vi "Doktorarbeit_Cornelius_1.73.vi"(0 "Heizer":refnum<visa-resource-name>="COM1", 1 "Setpoint\n START":bool, 2 "Write to File":bool, 3 "SP 1 shall be (°C)":dbl=20.0 min=0.0 max=999.0, 4 "Intervall (s)":u32=1 max=600, 5 "Write/\nRead":bool=TRUE, 6 "Delay (ms)":u32=500 min=100 max=600000, 7 "Auto Tune":bool, 9 "Standby":bool, 11 "Reset\nSTOPP":bool, 12 "Read Temperature":bool=TRUE, 13 "Get Values":bool, 15 "File Path":path) -> (8 "(°C)":dbl format="%#.3f", 14 "SP 1 is (°C)":dbl)   [LabVIEW 2010]
doc: "1. Verwendung\n\nDas Programm dient der Steuerung und Abfrage des Thermocontrollers I3252 und dem Auslesen von zwei VC 840 Messgeräten und einem Druckmessgerät Pfeiffer Single Gauge. \nDie Messgeräte werden Standardmäßig ausgelesen und erst nach Betätigung des Schalters \"Write to File\" in einer Textdatei abgespeichert. Das Eingabefeld \"Intervall\" legt den Abstand der Messpunkte fest.\nDer Setpoint für den Thermocontroller wird erst nach Betätigung des Tasters \"Setpoint START\" übernommen und angesteuert. Er wird ind den EEPROM des Gerätes geschrieben. Die Regelung kann mit Hilfe des Schalters \"Standby\" unterbrochen werden. Durch den Taster \"Reset STOPP\" kann der Setpoint aus dem EEPROM gelöscht werden.\nDie Eingabeflächen \"Constant\" und \"Thickness\" dienen der Berechnung des spezifischen Widerstands.\nDie Eingabeflächen \"User\" und \"Sample\" werden in den Header der Textdatei übernommen.\nDer Indikator \"File Path\" zeigt den aktuellen Speicherort der Textdatei an. Dieser wird nach ausschalten des Schalters \"Write to File\" gelöscht. Bei erneuten Schreiben muss ein neuer Speicherort gewählt werden. Bei Wahl desselben Speicherorts werden sämtliche bereits gespeicherte Daten gelöscht.\n\n\n2. Erläuterungen zum Blockdiagramm\n2.1 äußere Sequenz\nDie äußerte Sequenz besteht aus fünf Frames. Der erste dient der Initialisierung der Ports. Der zweite dient als Verzögerung um dem Programm genug Zeit zu geben die Ports zu öffnen. Jedoch senden die beiden VC 840 bereits Informationen an den Computer die in einem Puffer zwischengespeichert werden. Im dritten Frame wird dieser Puffer geleert. Somit kommt es zu keinem Framing Error. Desweiteren wird in diesem Frame die Startzeit der Messungen genommen. Im vierten Frame wird die eigentliche Messung und Verarbeitung der Daten durchgeführt. Die while-Schleife wird nur durch Auftreten eines Fehlers oder durch Betätigung des Stopbuttons auf dem Front Panel in der oberen linken Ecke unterbrochen. Im fünften und letzten Frame werden die Ports wieder geschlossen und beim Auftreten eines Fehlers wird das Programm automatisch gestoppt. Falls kein Fehler auftritt wird die Sequenz von vorne abgearbeitet.\n\n2.2 while-Schleife und innere Sequenz\n2.2.1 \"Event Structure\"\n2.2.1.1 Allgemein\nDer erste Frame beinhaltet ein \"Event Structure\". Dieser reagiert auf insgesamt elf verschiedene Ereignisse. Falls keines dieser Ereignisse auftreten sollte, warte die Struktur eine Millisekunde bevor die \"Event Structure\" verlassen wird. Die übrigen Ereignisse treten ein, wenn der entsprechende Kontroller eine Werteänderung erfährt.\n\n2.2.1.2 Event: Setpoint\nDieser Case besteht von außen nach innen aus einer Stacked Sequence, einer for-Loop und einer Flat Sequence die wiederum zwei \"Case Structures\" enthält. Als erstes wird bei dem Schalter \"Setpoint START\" der Blinkmodus aktiviert und bei dem Schalter \"Read Temperature\" deaktiviert. Danach folgt das eigentliche setzen des Temperatursollwerts. In der ersten Iteration wird dem Controller I3252 ein Schreibbefehl gesendet. Theoretisch kann der Setpoint in den RAM oder in den EEPROM geschrieben werden. Diese Auswahl erfolgt mit Hilfe des Schalters \"RAM\". Da das Schreiben in den RAM -Speicher aber aus diversen Gründen nicht erwünscht ist, wurde es nicht implementiert. Eine nachträgliche Implementierung ist aber leicht möglich, in dem die untere String-Konstante \"*P012\" durch \"*W012\" ersetzt wird. An diesem Befehl wird eine fünfstellige Hexadezimalzahl angehängt, die den Sollwert wiedergibt. Der Sollwert wird vorher mit zehn multipliziert, da das Komma standardmäßig nach der ersten Ziffer festgesetzt wurde (Bsp.: 800 wird gesendet um 80 einzustellen). Dieser Befehlsstrang wird an das Gerät mittels des SubVIs \"Comm_Interface\", auf welches später noch näher eingegangen wird, weitergegeben. Der durch das Gerät zurückgegebene String wird nicht verarbeitet.\nDie zweite Iteration dient dem Auslesen des eingestellten Sollwertes. Wahlweise kann der RAM- oder der EEPROM-Speicher ausgelesen werden. Die eigentliche Verarbeitung des Ausgabestrings erfolgt durch das SubVI \"Edit Setpoint\".\nDie Implementierung zur Einstellung des zweiten Setpoints erfolgt durch kopieren der ersten beiden Fälle und ersetzen der \"1\" im Befehf durch eine \"2\" (Bsp.: \"*P012\" zu \"*P022\"). Es darf aber nicht vergessen werden, dass dann ebenfalls die Anzahl der Iterationen angepasst werden muss.\nAls letztes wird der Blinkmodus des Schalters \"Setpoint START\" wieder deaktiviert.\n\n2.2.1.3 Event: Standby\nDieses Ereignis aktiviert bzw. deaktiviert als erstes den Blinckmodus des entsprechenden Schalters und sendet danach den Befehl zum aktivieren (\"*D03\") oder zum deaktivieren (\"*E03\") des Standbymodus an den Thermocontroller.\n\n2.2.1.4 Event: Set Command \nDer in das Feld \"Command shall be\" eingegebene Befehl wird an den Thermocontroller übermittlet. Die korrekte Form des Befehls ist im \"Communication Manuel\" nachzuschlagen. Das \"*\"-Zeichen wurde allerdings schon implementiert und muss somit nicht mit eingegeben werden.\n\n2.2.1.5 Event: Reset\nIn der ersten Iteration wird der Reset-Befehl an den Thermocontroller gesendet. In Folge wird der gesamte EEPROM-Speicher gelöscht. Deshalb wird in der zweiten Iteration der Setpoint aktualisiert. Dieser Befehl hat keinen Einfluss auf den RAM-Speicher. Die anschließende Wartezeit ist auf vier Sekunden festgesetzt und wurde empirisch ermittelt. Diese Zeit benötigt das Gerät um den Reset durchzuführen und für die Kommunikation wieder zur Verfügung zu stehen.\n\n2.2.1.6 Event: Auto Tune\nEs ist festgeschrieben, dass der Setpoint für die \"Auto Tune\"-Funktion wenigstens 20°C über der aktuellen Temperatur liegt. Deshalb wird zunächst der aktuelle Temperaturwert ausgelesen. Im zweiten Schritt werden zu diesem Wert zwanzig addiert und der Setpoint wird in den RAM-Speicher geschrieben. Das Schreiben in diesen Speicher ist nötig, da die \"Auto Tune\"-Funktion\" erst nach einem Reset startet. Im dritten Schritt wird der eigentliche Befehl für den \"Auto Tune\" gesendet (siehe dazu \"Communication Manuel\" S.27). Als vierte und letzte Iteration der for-Schleife folgt der bereits erwähnte Reset-Befehl. Der Temperatursollwert, der im RAM-Speicher eingetragen ist, muss zum Schluss wieder auf 0°C gesetzt werden. Die Zeit für die Ausführung des \"Auto Tune\"-Befehls wurde empirisch ermittelt und 45 s festgesetzt.\n\n2.2.1.7 Event: Write LOW/HI\nDieses Ereignis setzt die am Analogausgang anliegende Spannung fest. Normalerweise beträgt dieser Spannungswert 0-10 V. Das angeschlossene Netzteil verträgt aber maximal nur 2,3 V. Aus diesem Grund wird der \"%HIGH\" auf 23 gesetzt. Somit beträgt die maximal anliegende Spannung nur noch 23% von der maximal möglichen, d.h 2,3V. Ein niedrigerer Wert ist jederzeit möglich, genauso wie ein höherer für den Parameter \"%LOW\". Diese werden zunächst nacheinander in den RAM-Speicher geschrieben und anschließend wieder ausgelesen.\n\n2.2.1.8 Event: Set PID\nDie Werte für den PID-Regler können sowohl mit Hilfe der \"Auto Tune\"-Funktion, als auch manuell eingestellt werden. Es wird wiederum zwischen dem Schreiben in den RAM- und dem EEPROM-Speicher unterschieden. Zunächst werden die Werte für \"P\", \"I\" und \"D\", in dieser Reihenfolge, gesetzt und danach die aktuellen Werte ausgelesen.\n\n2.2.1.9 Event: Get Values\nDieses Ereignis hat zur Folge, dass die Werte für \"P\", \"I\", \"D\", \"%LOW\", \"%HIGH\" und des Setpoints wahlweise aus dem RAM- oder EEPROM-Speicher gelesen werden. Die aktuellen Werte werden nicht nur in die entsprechenden Anzeigefelder übernommen, sondern auch in die entsprechenden Eingabefelder, mit Ausnahme des Temperatursollwerts. \n\n2.2.1.10 Event: RAM\nPrinzipiell kann zwischen dem Schreiben in den RAM- oder EEPROM-Speicher des Thermocontrollers gewählt werden. Die entsprechende Schalterposition auf dem Frontpanel zeigt den aktuell verwendeten Speicher an. Die Anzeigewerte werden bei jedem Umschalten aktualisiert und sind im entsprechenden Speicher eingetragen. Die Implementierung ist identisch mit der des Ereignisses \"Get Values\". Es gilt zu beachten, dass die Werte für \"%LOW\" und \"%HIGH\" nur in den RAM-Speicher geschrieben werden können und somit auch nur aus diesem ausgelesen werden können.\n\n2.2.1.11 Event: Set Gauge to Zero\nMit Hilfe der SubVIs \"Get Pressure\" und \"Offset Display\" werden die Werte für den alten und den neuen Offset und der durch den zweiten Drucksensor ermittelt Druck ermittelt. \n\n2.2.1.12 Event: Write to File\nSollte der Schalter \"Write to File\" aktiviert werden, d.h. Schalterposition oben, so wird zunächst durch das SubVI \"Header\" ein Header für die unter \"File Path\" definierte Datei angelegt. Alle Werte, die bereits in der entsprechenden Datei stehen, werden dabei gelöscht.\n\n2.2.2 \"Timed Structures\"\nIm dritten Frame der inneren Sequenz werden die Werte für Zeitpunkt, Temperatur, Spannung, Strom und Druck ermittelt. Damit die Werte zum gleichen Zeitpunkt aufgenommen werden, werden \"Timed Sequences\" eingesetzt. Mit dem entsprechenden Schalter auf dem Front Panel unter dem Tab \"Settings\" kann gewählt werden, ob das entsprechende Gerät ausgelesen werden soll oder nicht. Die einzelnen Sequenzen werden parallel abgearbeitet, womit die Prozesszeit von diesem Frame durch der zeitintensivsten Sequenz abhängt. Dies ist in aller Regel das Auslesen der Temperatur, da ein \"Delay\" von 500 ms oder größer benötigt wird, um den Controller ordentlich ansprechen zu können.\nDie Systemzeit wird durch das SubVI \"System Time in Seconds\" in Sekunden umgerechnet und der in dem Parameter \"Starttime\" gespeicherte Wert wird abgezogen. Somit werden die Sekunden seit dem Start des Programms gezählt.\n\n2.2.3 restlichen Frames\nIm zweiten Frame wird das Intervall zwischen den einzelnen Messwerten festgelegt. Dabei wird der Wert des Parameters \"Delay\" abgezogen. Dieser Wert beträgt im Normalfall 500 ms und ist somit nicht vernachlääsigbar.\nDer Vierte Frame beinhaltet die Umrechnung des Temperatur-Strings in einen Temperaturwert durch das SubVI \"Edit Tmperature\", die Berechnung des spezifischen Widerstands durch das SubVI \"Resistivity Calculation\" und die Überprüfung des Druckwerts. Auch werden die neu gewonnen Werte in das entsprechende Shift-Register übernommen. Falls der Druckwert einen in dem Parameter \"Pressure Limit (mbar)\" festgelegten Grenzwert überschreiten sollte, wird der Thermocontroller automatisch in den Standby-Modus versetzt. Des Weiteren wird der Schalter \"Standby\" solange gesperrt, wie der Druck oberhalb des Grenzwertes liegt. Wenn der Druck wieder unter den Grenzwert gesunken ist, wird der Standby-Befehl nicht automatisch aufgehoben, sondern muss vom Benutzer durch Betätigung des entsprechenden Schalters gegeben werden.\nIm fünften Frame werden die Diagramme erstellt. Dabei wird jedes Mal von neuem das gesamte Shift-Register als Graph dargestellt. Weiterhin werden die Messwerte in ein 1D-Array geschrieben.\nDer sechste und letzte Frame beinhaltet den eigentlich Schreibvorgang der Messwerte in eine Textdatei und die Überprüfung ob ein Fehler vorliegt.\n\n2.3 SubVIs\n2.3.1 Allgemein\nDie SubVIs für die Messgeräte VC840 und das Druckmessgerät wurden aus anderen Quellen übernommen. \n\n2.3.2 \"Header\"\nIn den Header wird zunächst das aktuelle Datum und die aktuelle Zeit übernommen. Die ausgewählte Datei wird dabei überschrieben. Danach wird der Name des Benutzers und der Probe übernommen. Zum Schluss werden die Einheiten in einer Reihe, durch einen Tabulator getrennt, in den Header geschrieben.\n\n2.3.3 \"I3252 Comm Interface\"\nDieses VI stellt die Kommunikation mit dem Thermocontroller her und gibt den Ausgabe-String zurück.\n\n2.3.4 \"I3252 Edit Setpoint\"\nIm Ausgabe-String vom Thermocontroller ist an der vierten Stelle die Stelle des Dezimalpunktes verschlüsselt. Dieses Hexadezimalzahl wird herausgefiltert und an ein \"ENUM Controller\" übergeben. Dieser weist der Hexadezimalzahl eine Nummer zu, mit welcher ein Wert aus einem Array entnommen wird. Dieser Wert dient als Quotient. Der tatsächliche Wert kann somit errechnet werden.\n\n2.3.5 \"I3252 Edit Temperature\"\nDer Temperatur-String, der vom Thermocontroller zurückgegeben wird, wird in eine Dezimalzahl umgewandelt. Manchmal kommt es aus zu Dropouts, die durch dieses Programm herausgefiltert werden. Der letzte Wert wird dabei in einer \"Feedback Node\" gehalten unter der Annahme, dass sich der Temperaturwert nicht sprunghaft ändert.\n\n2.3.6 \"Resistivity Calculation\"\nDer spezifische Widerstand wird nach folgender Formel ausgerechnet. Dabei entspricht t der Dicke der Probe und C ist eine Konstante.\nrho=C*pi*t*U/(ln( 2)*I)\n\n2.3.7 \"System Time in Seconds\"\nZunächst wird die aktuelle Systemzeit ausgelesen. Danach wird diese in Stunden, Minuten und Sekunden aufgeteilt, alles in Sekunden umgerechnet und letztendlich addiert."
uses:
  <vilib>/Platform/TimedLoop/XDataNode/XDataNode.xnode
  <vilib>/Platform/TimedLoop/XDataNode/timing_clust.ctl
  <vilib>/Platform/TimedLoop/XDataNode/nitl_modes.ctl
  <vilib>/Platform/TimedLoop/XDataNode/wakeup.ctl
  <vilib>/Instr/_visa.llb/VISA Configure Serial Port (Instr).vi
  <vilib>/Platform/TimedLoop/scheduler/LVUserAPI/_suppVIs/Create_1kHz_TSource.vi
  <vilib>/Utility/file.llb/Write To Spreadsheet File (DBL).vi
  <vilib>/Platform/TimedLoop/XDataNode/XDNodeRunTimeDep.lvlib
  Labview 8 Tutorial/Dual Gauge/Dual Gauge.lvlib
panel:
  out "appended array":dbl[](array[numeric])
  in  "Tab Control":T1(tab)
  out "Pirani (VVP1 Scroll)":cluster{dbl[], dbl[]}(graph)
  in  "Thickness (nm)":dbl min=0.0
  in  "Constant":dbl=4.532 min=0.0 max=5.0
  in  "Sample":string
  in  "User":string
  out "Thermocouple (Sample holder 1)":cluster{dbl[], dbl[]}(graph)
  out "current time (s)":dbl
  out "data logger intervall (s)":dbl
  out "loop time (s)":dbl
  in  "stop":bool
  out "CMR275 Baratron":cluster{dbl[], dbl[]}(graph)
  out "Pressure Baratron 2":dbl format="%#_4e"
  out "PKR251 FullRange":cluster{dbl[], dbl[]}(graph)
  out "Pressure FullRange 2":dbl format="%#_3e"
  out "Pressure Pirani 2":dbl format="%#_3e"
  out "Pressure OpenPort":cluster{dbl[], dbl[]}(graph)
  out "Pressure OpenPort2":dbl caption="current"
  out "Current Baratron (mbar)":dbl
  out "Error COM6 Out":cluster{"status":bool, "code":i32} caption="Cluster (Ausgang)"
  out "Pressure Pirani":dbl format="%.3e"
  out "Pressure OpenPort":dbl format="%.3e"
  out "Status Sensor 4":i32(ring) items=["data OK", "underrange", "overrange", "sensor error", "sensor off", "no sensor", "ID error"]
  out "Status Pirani":i32(ring) items=["data OK", "underrange", "overrange", "sensor error", "sensor off", "no sensor", "ID error"]
  in  "COM6 in":refnum<visa-resource-name>="COM6"
  out "Error COM5 Out":cluster{"status":bool, "code":i32} caption="Cluster (Ausgang)"
  out "Pressure FullRange":dbl format="%.3e"
  out "Pressure Baratron":dbl format="%.3e"
  out "Status FullRange":i32(ring) items=["data OK", "underrange", "overrange", "sensor error", "sensor off", "no sensor", "ID error"]
  out "Status Baratron":i32(ring) items=["data OK", "underrange", "overrange", "sensor error", "sensor off", "no sensor", "ID error"]
  in  "COM5 in":refnum<visa-resource-name>="COM5"
  out "Error Out":bool
  in  "Set Gauge to Zero":bool
  in  "Pressure Limit (mbar)":dbl=1.0 min=0.0 max=1100.0
  out "Current Offset (mbar)":dbl
  out "Old Offset (mbar)":dbl
  out "Pressure 2 (mbar)":dbl
  in  "VC 840 2":refnum<visa-resource-name>="COM7"
  out "Reading 2":dbl format="%_4f"
  out "Mode 2":enum16{"?", "Diode", "Beep", "DC", "AC"}(ring)
  out "Unit 2":string
  in  "VC 840 1":refnum<visa-resource-name>="COM7"
  out "Reading 1":dbl format="%_4f"
  out "Mode 1":enum16{"?", "Diode", "Beep", "DC", "AC"}(ring)
  out "Unit 1":string
  out "Status 1":T2
  out "Status 2":T2
  in  "Read VC 840 1":bool
  in  "Read VC 840 2":bool
  in  "Set Command":bool
  in  "Set PID":bool
  in  "Write LOW/HI":bool
  out "% HIGH is":u32
  out "% LOW is":u32
  in  "% High shall be":u32=23 max=24
  in  "% LOW shall be":u32 max=25
  in  "Flow Control":u16(ring) items=["None"=0, "XON/XOFF"=1, "RTS/CTS"=2, "DTR/DSR"=4]
  in  "Stop Bits":u16(ring)=10 items=["1.0"=10, "1.5"=15, "2.0"=20]
  in  "Parity":u16(ring)=1 items=["None", "Odd", "Even", "Mark", "Space"]
  in  "Data Bits":u16=7 min=5 max=8 step=1
  in  "Baud Rate":u32=9600
  out "Command is":string
  in  "Command shall be":string
  in  "RAM":bool=TRUE caption="EEPROM"
  out "D (Rate) is":u32
  out "I ( Reset1) is":u32
  out "P (PB1) is":u32
  in  "D (Rate) shall be":u32 max=3999
  in  "I ( Reset1) shall be":u32 max=3999
  in  "P (PB1) shall be":u32 max=9999
  in  "Read Pressure":bool=TRUE
  out "Current":cluster{dbl[], dbl[]}(graph)
  out "Voltage":cluster{dbl[], dbl[]}(graph)
  out "Voltage (V)":dbl format="%.4e"
  out "Current (A)":dbl format="%.4e"
  out "Resistivity":cluster{dbl[], dbl[]}(graph)
  out "Resistivity (Ohm*cm)":dbl format="%.3e"
  # "°C"
  # "mbar"
  # "mbar"
  # "mbar"
  # "mbar"
  # "Offset Control"
  # "Sensor Diagnose"
  # "mbar"
  # "mbar"
  # "mbar"
  # "mbar"
  # "VC 840 Control"
  # "I3252 Control"
  # "Pfeiffer Control"
  # "Authors:  Daniel Schuster (sir-dan@web.de)\n                 Steffen Cornelius (s.cornelius@hzdr.de)\n                 Nico Spahn (x)\n\n                 premade SubVIs for readout of Pfeiffer gauge and VC840 Multimeters were used\n                 SubVI \"I3252_Comm_Interface\" is based on a modified Labview example\n\nRelease:  v1.0    \n\nVersion History:\n\nv1.1  -    28.06.2011\n             - Format des Files geändert von %.3f auf %g\n             - maximale Eingabewerte für PID begrenzt\nv1.2  -    12.07.2011\n             - Anzeige p,rho, U, V auf Scientific geändert\n             - y-Achse p,rho auf Log geändert\n             - numerische Zeitanzeige hinzugefügt\n             - 4PP Constant: pi/ln(2)=4,532 set as the default value\nv1.3  -    25.07.2011\n             - Zeitvariable auf EXT geändert, um Sprünge in Diagrammen loszuwerden\nv1.4  -   27.07.2011\n             - ALLE Variablen auf DBL zurückgesetzt wegen Formatierungsproblem im File\n             - Zeitberechnung neu gemacht (Tick count differenzen) -> Zeitsprünge korrigiert ?\n             - Delay/Intervall überarbeitet\nv1.5  -   05.12.2012\n                - Austausch der alten Pfeifer SubvIs durch neue -> nun alle 4 Kanäle des DualGauge\n                                                                                                         Controllers gleichzeitig auslesbar\n                - neue Pfeiffer SubVIs verwendet in Druckwertauslesung und Offset Berechnung des Baratron\n                  Druckes (COM5 Sensor1)\n                - Neuarragement des GUI -> FullRange und Baratron neben Temperatur auf Haupseite zu sehen\n                                                                   Pirani und OpenPort auf Meas.2 zu sehen\n                                                                   Diagnose Seite umfasst nun auch Widerstandsdiagramm\n                - Änderungen der Settingseite -> nun alle 4 Drucksensoren mit aktuellem Messwert und Gerätestatus\n                                                                           zu sehen\n                - The readout of the PID-Temperature Controller and the VC840 Multimeters was not modified\nv1.73  -  18.10.2013\n                - Layout Änderungen"
  # "Version 1.73    - last change 18.10.2013"
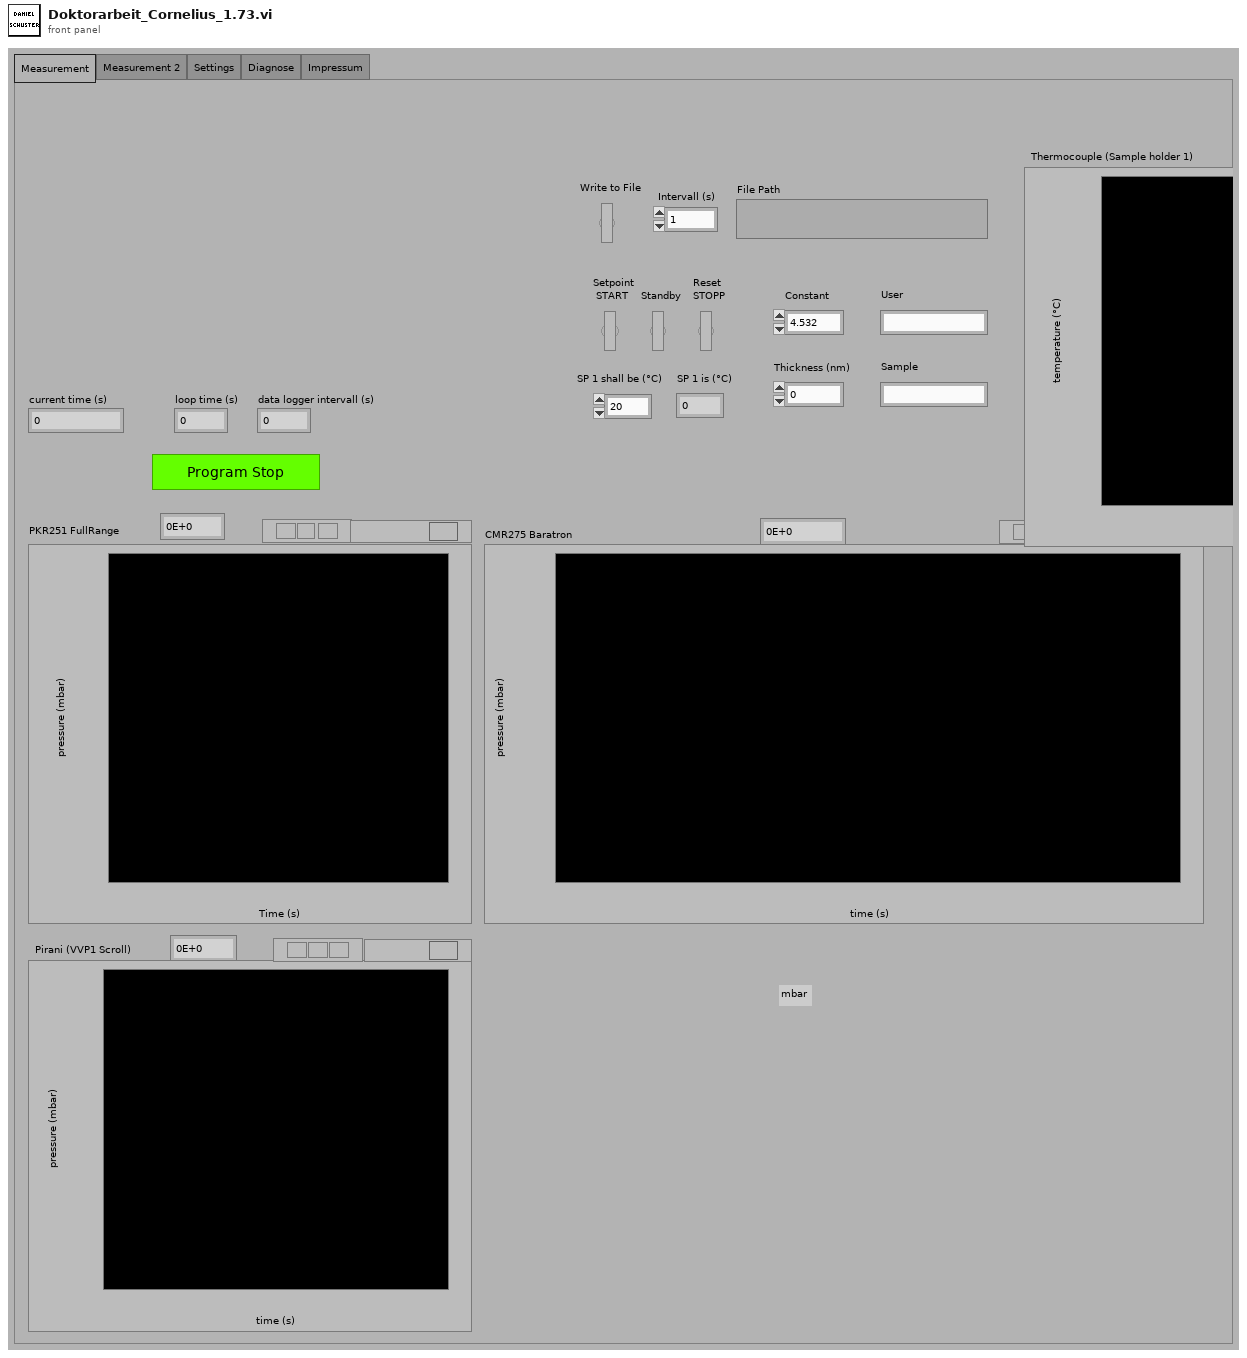
[diagram p1: front panel]
types:
  T1 = enum32{"Measurement", "Measurement 2", "Settings", "Diagnose", "Impressum"}
  T2 = cluster{"Low Bat":bool, "Auto":bool, "Delta":bool, "Hold":bool, "RS232":bool}
  T3 = typedef "XDNodeRunTimeDep.lvlib/timing_clust.ctl" = cluster{"Expected End [f-1]":u64, "Actual End [f-1]":u64, "Finished Late? [f-1]":bool, "Expected End [i-1]":u64, "Actual End [i-1]":u64, "Finished Late? [i-1]":bool, "Expected Start [i]":u64, "Actual Start [i]":u64, "Expected Start [f]":u64, "Actual Start [f]":u64, "Source Name":string, "Structure Name":string, "Period":i64, "Deadline":i64, "Offset":i64, "Start":i64, "Priority":i32, "Timeout":i32, "Mode":T4, "Wakeup Reason":T5, "Error":errorcluster, "Source Type":string, "Secondary Source Type":string, "Global End Time":u64, "Global Start Time":u64, "Frame Duration":u64, "Iteration Duration":u64, "Assigned CPU":i32, "I/O Scan Engine Mode":u32}
  T4 = typedef "XDNodeRunTimeDep.lvlib/nitl_modes.ctl" = enum32{"No Change", "Process missed periods, maintain original phase", "Discard missed periods, maintain original phase", "Process missed periods, ignore original phase", "Discard missed periods, ignore original phase"}
  T5 = typedef "XDNodeRunTimeDep.lvlib/wakeup.ctl" = enum32{"Normal", "Aborted", "Asynchronous wakeup", "Timing source error", "Timed loop error", "Timeout"}
  T6 = enum8{"Enabled", "Disabled", "Disabled and Grayed Out"}
  T7 = cluster{"VISA resource name out":refnum<visa-resource-name>, "error out":errorcluster, "Delay (ms)":u32, "Write/\nRead":bool}
  T8 = cluster{"Pressure":dbl, "Pressure":dbl, "Pressure":dbl, "Pressure":dbl}
  T9 = cluster{"COM5 in":refnum<visa-resource-name>, "error out":errorcluster, "COM6 in":refnum<visa-resource-name>, "error out":errorcluster}
  T10 = cluster{"COM5 out":refnum<visa-resource-name>, "Cluster (Ausgang)":errorcluster, "COM6 out":refnum<visa-resource-name>, "Cluster (Ausgang) 2":errorcluster}
  T11 = cluster{"Pressure Baratron":dbl, "Pressure FullRange":dbl, "Pressure Pirani":dbl, "Pressure Sensor 4":dbl}
  T12 = cluster{"COM5 out":refnum<visa-resource-name>, "error out":errorcluster, "COM6 out":refnum<visa-resource-name>, "error out":errorcluster}
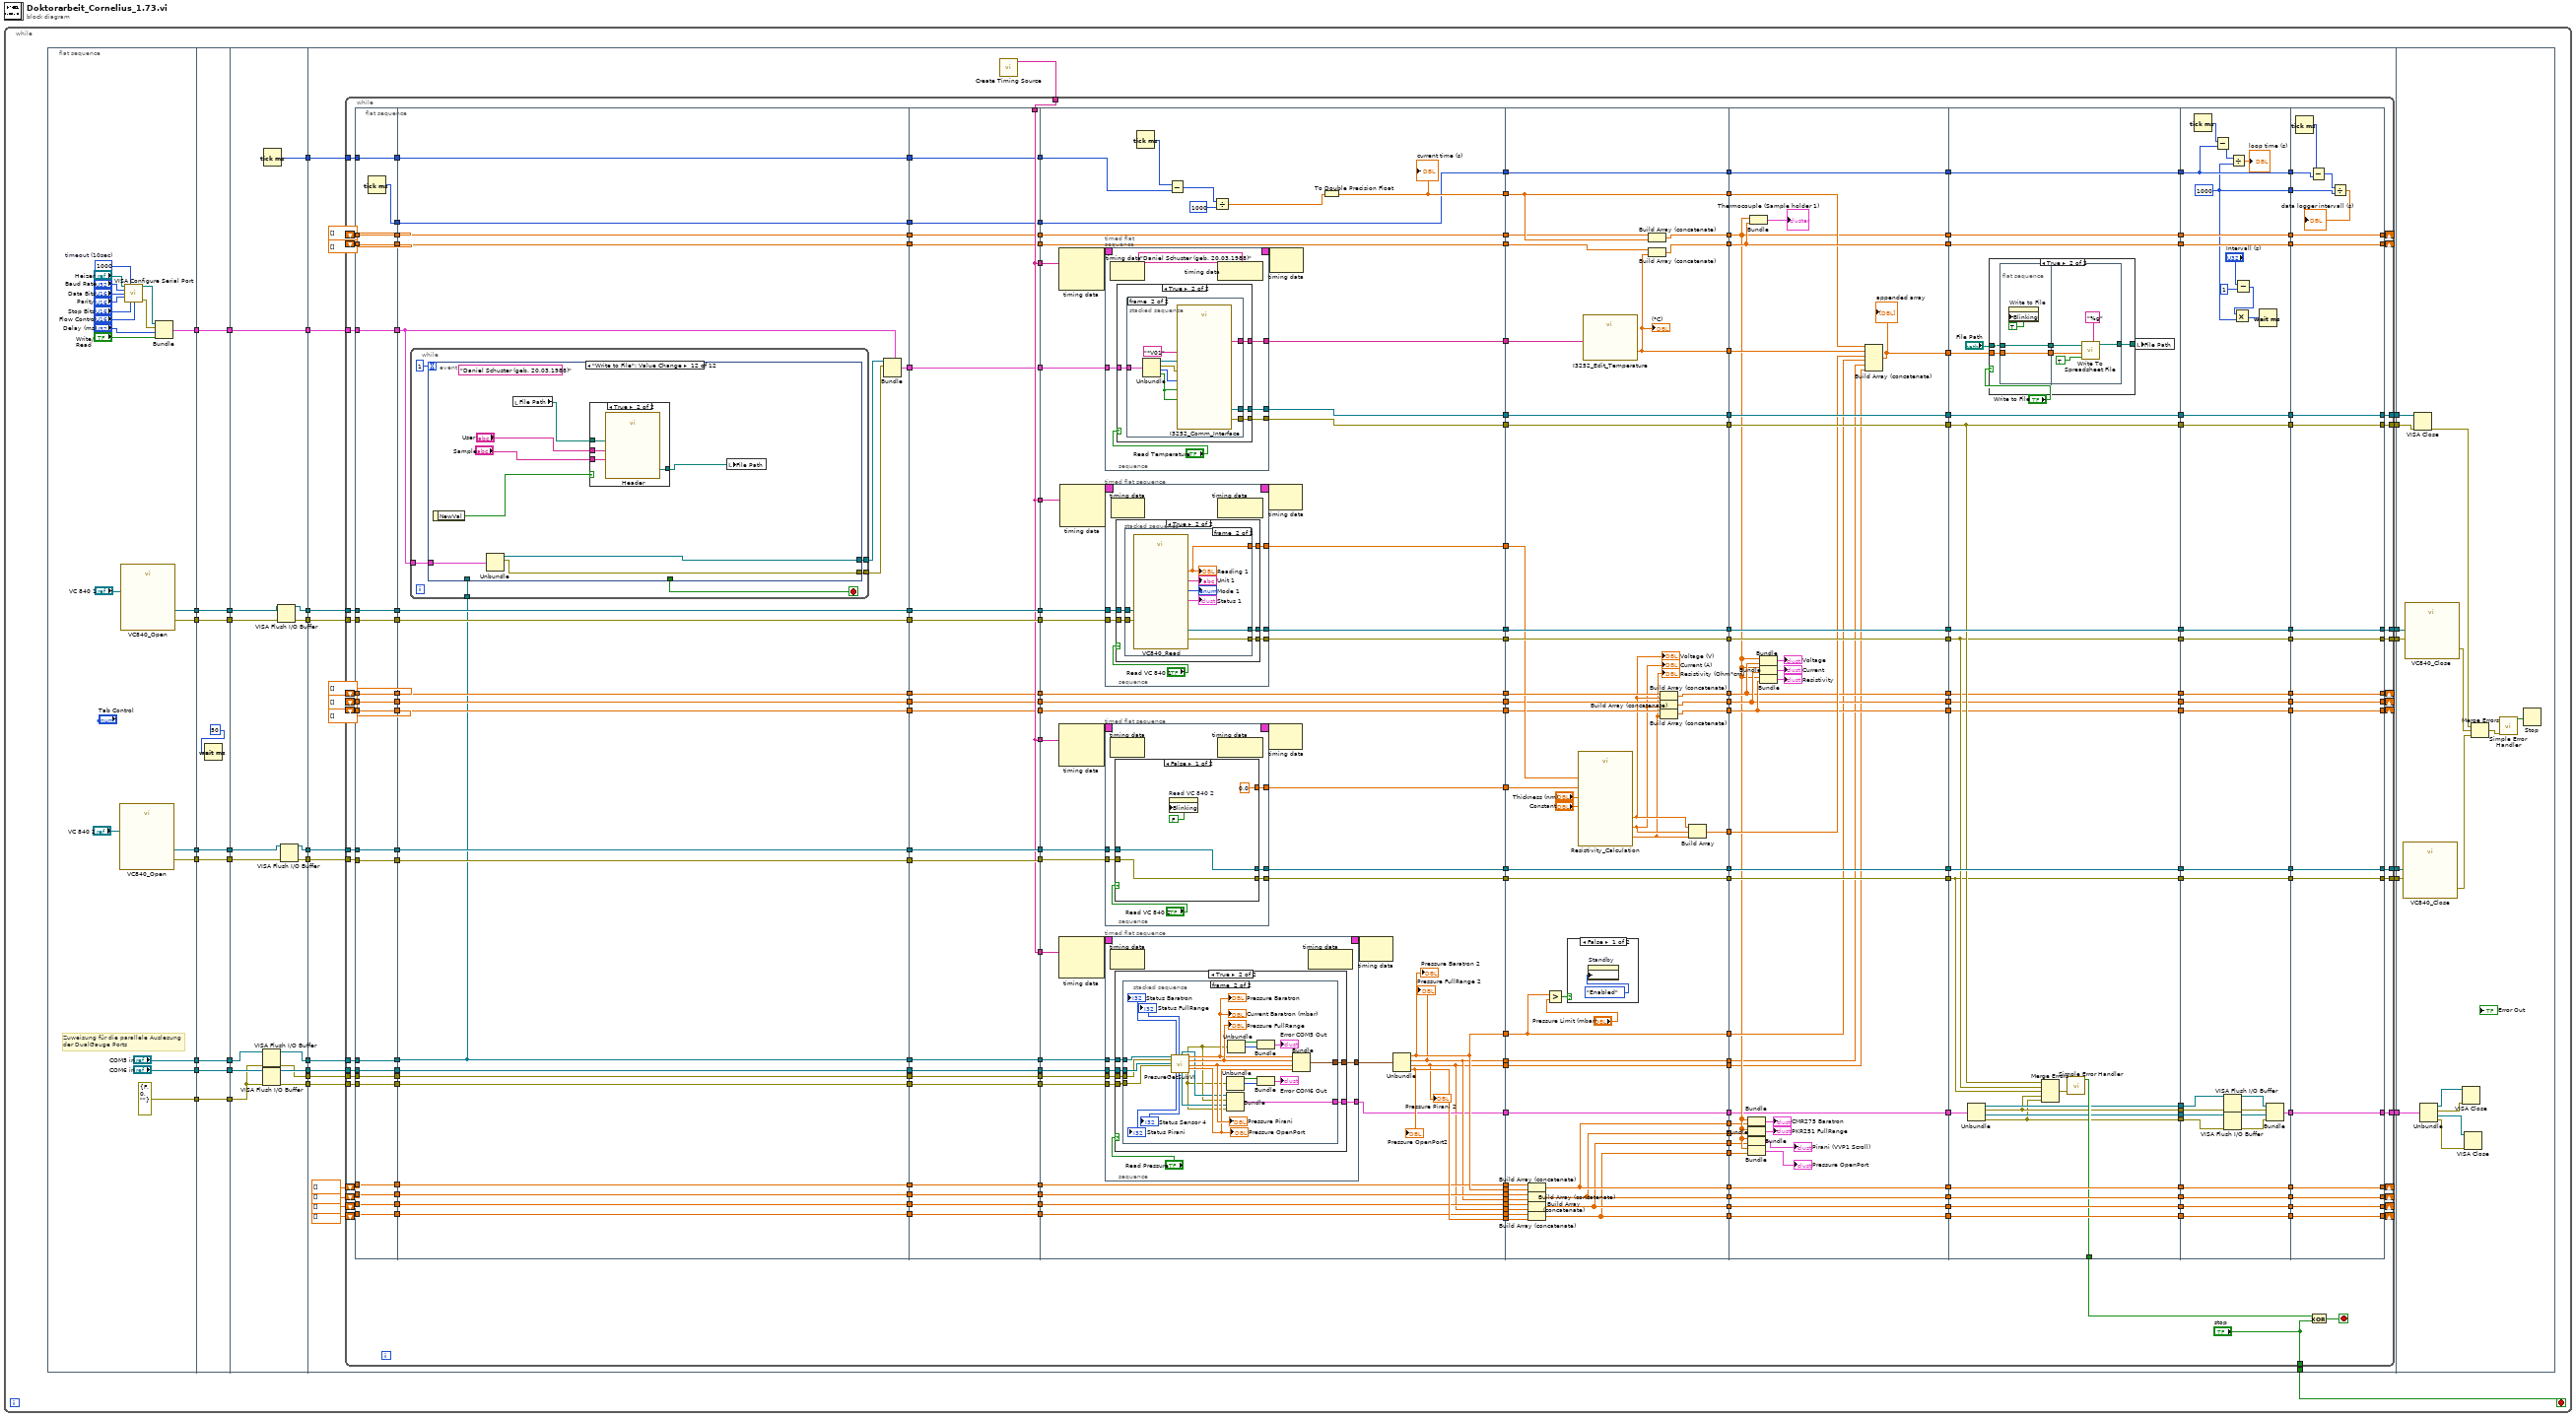
[diagram p0: block diagram]
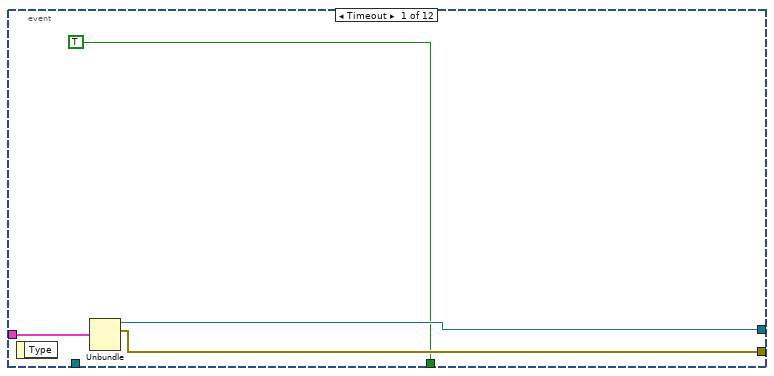
[diagram p2: hidden frame]
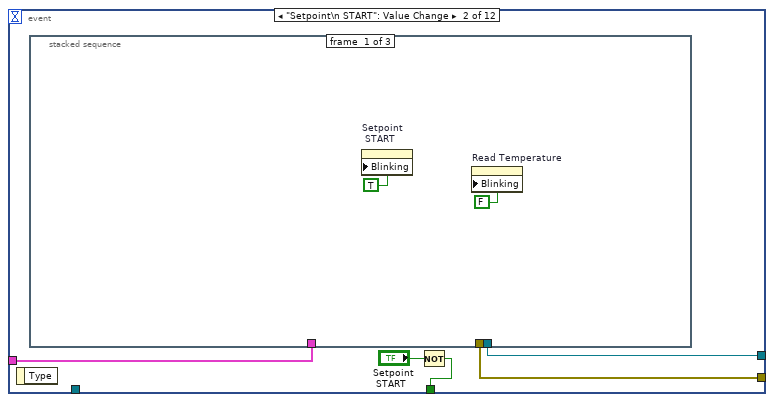
[diagram p3: hidden frame]
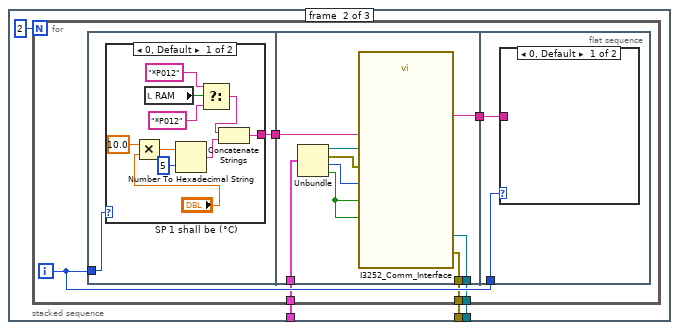
[diagram p4: hidden frame]
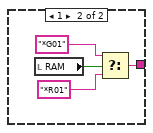
[diagram p5: hidden frame]
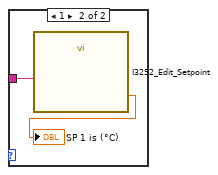
[diagram p6: hidden frame]
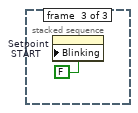
[diagram p7: hidden frame]
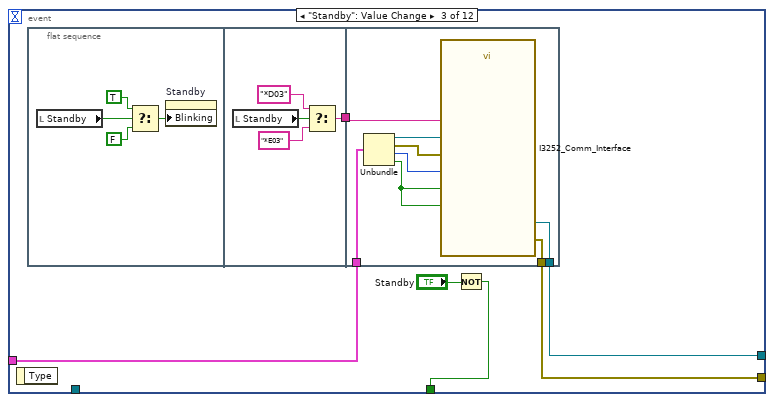
[diagram p8: hidden frame]
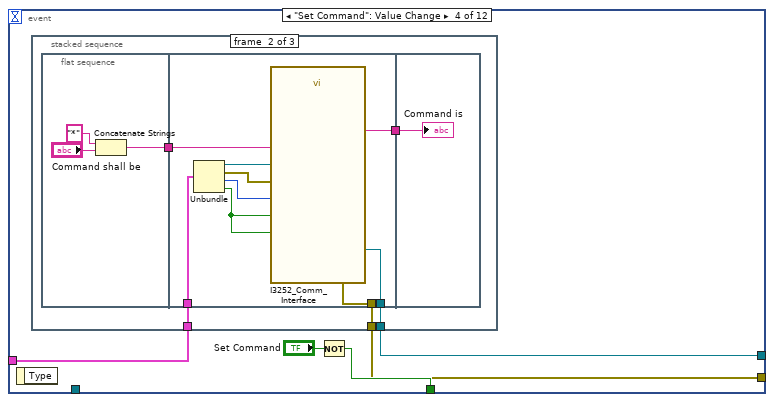
[diagram p9: hidden frame]
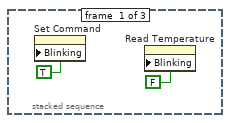
[diagram p10: hidden frame]
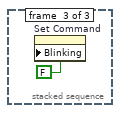
[diagram p11: hidden frame]
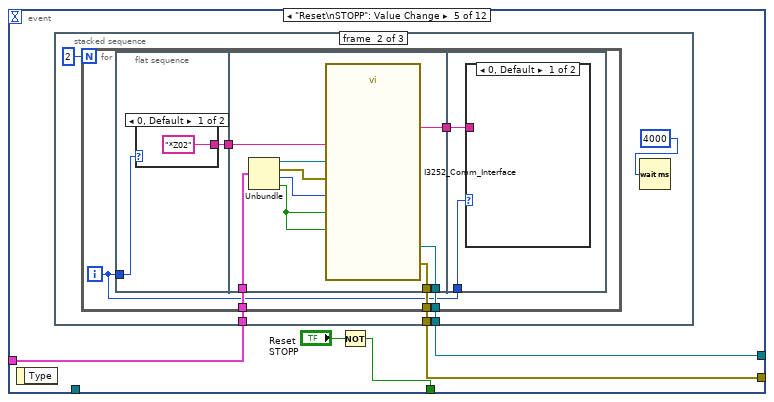
[diagram p12: hidden frame]
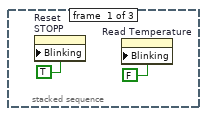
[diagram p13: hidden frame]
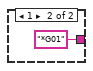
[diagram p14: hidden frame]
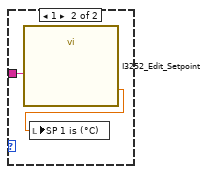
[diagram p15: hidden frame]
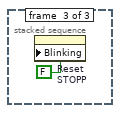
[diagram p16: hidden frame]
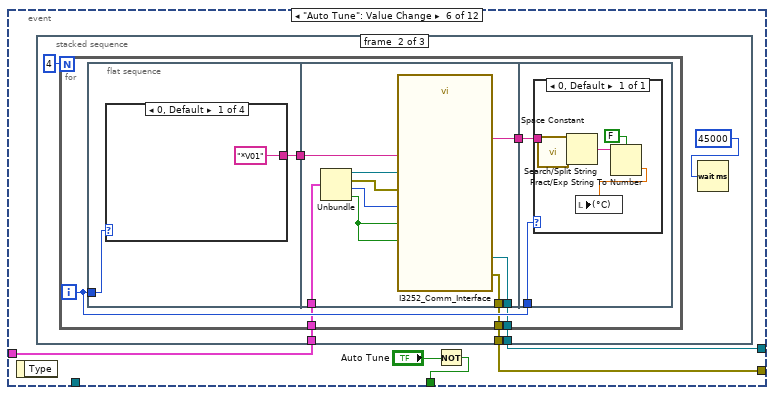
[diagram p17: hidden frame]
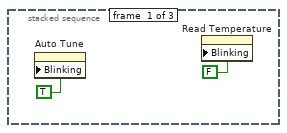
[diagram p18: hidden frame]
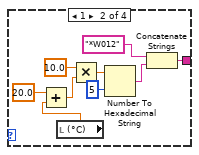
[diagram p19: hidden frame]
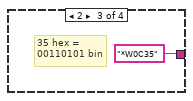
[diagram p20: hidden frame]
diagram:
  n1 = while {
    stop <- w6 stop-if-true
    n2 = flat-sequence {
      tunnel: [w54] -> w34
      tunnel: [w55] -> w33
      tunnel: [w40] -> w32
      tunnel: [w53] -> w31
      tunnel: [w52] -> w30
      tunnel: ["COM5 in"] -> w29
      tunnel: ["COM6 in"] -> w28
      tunnel: [errorcluster {"status"=FALSE, "code"=0, "source"=""} ("Fehler (Eingang)")] -> w3
      tunnel: w34 -> [w64]
      tunnel: [w64] -> w27
      tunnel: w33 -> [w63]
      tunnel: [w63] -> w26
      tunnel: w32 -> [w62]
      tunnel: [w62] -> w25
      tunnel: w31 -> [w61]
      tunnel: [w61] -> w24
      tunnel: w30 -> [w60]
      tunnel: [w60] -> w23
      tunnel: [w58] -> w22
      tunnel: w29 -> [w58]
      tunnel: [w57] -> w21
      tunnel: w28 -> [w57]
      tunnel: [w56] -> w4
      tunnel: w3 -> [w56]
      tunnel: w27 -> [w75]
      tunnel: [w74] -> w20
      tunnel: w26 -> [w76]
      tunnel: [w73] -> w19
      tunnel: w25 -> [w81]
      tunnel: [w81] -> w18
      tunnel: w24 -> [w78]
      tunnel: [w79] -> w17
      tunnel: w23 -> [w77]
      tunnel: [w80] -> w16
      tunnel: [w72] -> w15
      tunnel: [w70] -> w14
      tunnel: w22 -> [w71]
      tunnel: [w69] -> w13
      tunnel: w21 -> [w68]
      tunnel: w4 -> [w67]
      tunnel: [w66] -> w2
      tunnel: [w65] -> w1
      tunnel: w20 -> [w109]
      tunnel: w19 -> [w108]
      tunnel: w18 -> [w107]
      tunnel: w17 -> [w105]
      tunnel: w16 -> [w104]
      tunnel: [w103] -> w12
      tunnel: [w102] -> w11
      tunnel: [w101] -> w10
      tunnel: [w100] -> w9
      tunnel: [w99] -> w8
      tunnel: [w98] -> w7
      tunnel: w15 -> [w92]
      tunnel: w14 -> [w91]
      tunnel: w13 -> [w90]
      tunnel: [w85] -> w6
      tunnel: [w84] -> w5
      tunnel: w2 -> [w83]
      tunnel: w1 -> [w82]
      tunnel: w12 -> [w1292]
      tunnel: w11 -> [w1291]
      tunnel: w10 -> [w1294]
      tunnel: w9 -> [w1293]
      tunnel: w8 -> [w1296]
      tunnel: w7 -> [w1295]
      tunnel: w5 -> [w1289]
      frame #0 {
        w41 = u32 1000  # timeout (10sec)
        # "Zuweisung für die parallele Auslesung\nder DualGauge Ports"
        n3 = call "VC840_Open.vi"("VISA resource name"="VC 840 2") -> ("error out"=w52:errorcluster, "VISA resource name out"=w53:refnum<visa-resource-name>)  [unwired: 1 in, 8 out]
        n4 = call "VC840_Open.vi"("VISA resource name"="VC 840 1") -> ("error out"=w55:errorcluster, "VISA resource name out"=w54:refnum<visa-resource-name>)  [unwired: 1 in, 8 out]
        n5 = call-poly "VISA Configure Serial Port"("VISA resource name"="Heizer", "timeout (10sec)"=w41, "baud rate (9600)"="Baud Rate", "data bits (8)"="Data Bits", "parity (0:none)"="Parity", "stop bits (10: 1 bit)"="Stop Bits", "flow control (0:none)"="Flow Control") -> ("VISA resource name out"=w50:refnum<visa-resource-name>, "error out"=w51:errorcluster)  [unwired: 2 in, 5 out]
        n6 = Bundle("VISA resource name out"=w50, "error out"=w51, "Delay (ms)"="Delay (ms)", "Write/\nRead"="Write/\nRead") -> (w40:T7)  [unwired: 1 in]
      }
      frame #1 {
        n7 = Wait (ms)(milliseconds to wait=u32 50) -> ()  [unwired: 1 out]
      }
      frame #2 {
        n8 = VISA Flush I/O Buffer(VISA resource name=w71, error in (no error)=w67) -> (VISA resource name out=w70:refnum<visa-resource-name>, error out=w66:errorcluster)  [unwired: 1 in]
        n9 = VISA Flush I/O Buffer(VISA resource name=w68, error in (no error)=w67) -> (VISA resource name out=w69:refnum<visa-resource-name>, error out=w65:errorcluster)  [unwired: 1 in]
        n10 = Tick Count (ms)() -> (millisecond timer value=w72:u32)
        n11 = VISA Flush I/O Buffer(VISA resource name=w75, error in (no error)=w76) -> (VISA resource name out=w74:refnum<visa-resource-name>, error out=w73:errorcluster)  [unwired: 1 in]
        n12 = VISA Flush I/O Buffer(VISA resource name=w78, error in (no error)=w77) -> (VISA resource name out=w79:refnum<visa-resource-name>, error out=w80:errorcluster)  [unwired: 1 in]
      }
      frame #3 {
        n13 = call-poly <vilib>:"Create Timing Source.vi"() -> ("name (out)"=w106:string)  [unwired: 10 in, 1 out]
        n14 = while {
          tunnel: w109 -> [w323]
          tunnel: w108 -> [w322]
          tunnel: w107 -> [w321]
          tunnel: w106 -> [w314]
          tunnel: w105 -> [w307]
          tunnel: w104 -> [w306]
          tunnel: [w302] -> w103
          tunnel: [w301] -> w102
          tunnel: [w299] -> w101
          tunnel: [w297] -> w100
          tunnel: [w295] -> w99
          tunnel: [w293] -> w98
          shift-right: [w266] -> _
          shift-left: dbl[] [] -> [w271]
          shift-right: [w244] -> _
          shift-left: dbl[] [] -> [w279]
          shift-right: [w268] -> _
          shift-left: dbl[] [] -> [w275]
          shift-right: [w241] -> _
          shift-left: dbl[] [] -> [w278]
          shift-right: [w238] -> _
          shift-left: dbl[] [] -> [w277]
          tunnel: w92 -> [w232]
          tunnel: w91 -> [w188]
          tunnel: w90 -> [w184]
          shift-right: [w140] -> _
          shift-left: dbl[] [] -> [w170]
          shift-right: [w138] -> _
          shift-left: dbl[] [] -> [w168]
          shift-right: [w136] -> _
          shift-left: dbl[] [] -> [w166]
          shift-right: [w134] -> _
          shift-left: dbl[] [] -> [w164]
          tunnel: ["stop"] -> w85
          tunnel: [w126] -> w84
          tunnel: w83 -> [w121]
          tunnel: w82 -> [w119]
          stop <- w125 stop-if-true
          n15 = flat-sequence {
            tunnel: w232 -> [w333]
            tunnel: w271 -> [w334]
            tunnel: w275 -> [w335]
            tunnel: w277 -> [w336]
            tunnel: w278 -> [w337]
            tunnel: w279 -> [w338]
            tunnel: w306 -> [w339]
            tunnel: w307 -> [w340]
            tunnel: w321 -> [w341]
            tunnel: w322 -> [w342]
            tunnel: w323 -> [w343]
            tunnel: [w343] -> w231
            tunnel: [w342] -> w230
            tunnel: [w341] -> w229
            tunnel: [w340] -> w228
            tunnel: [w339] -> w227
            tunnel: [w338] -> w226
            tunnel: [w337] -> w225
            tunnel: [w336] -> w224
            tunnel: [w335] -> w223
            tunnel: [w334] -> w222
            tunnel: [w333] -> w221
            tunnel: [w332] -> w203
            tunnel: [w331] -> w189
            tunnel: w188 -> [w331]
            tunnel: [w330] -> w185
            tunnel: w184 -> [w330]
            tunnel: [w329] -> w171
            tunnel: w170 -> [w329]
            tunnel: [w328] -> w169
            tunnel: w168 -> [w328]
            tunnel: [w327] -> w167
            tunnel: w166 -> [w327]
            tunnel: [w326] -> w165
            tunnel: w164 -> [w326]
            tunnel: [w325] -> w122
            tunnel: w121 -> [w325]
            tunnel: [w324] -> w120
            tunnel: w119 -> [w324]
            tunnel: [w366] -> w320
            tunnel: [w365] -> w318
            tunnel: [w361] -> w316
            tunnel: [w360] -> w311
            tunnel: [w359] -> w309
            tunnel: [w358] -> w276
            tunnel: [w357] -> w272
            tunnel: [w356] -> w252
            tunnel: [w355] -> w249
            tunnel: [w354] -> w247
            tunnel: [w353] -> w233
            tunnel: w231 -> [w366]
            tunnel: w230 -> [w365]
            tunnel: w229 -> [w364]
            tunnel: w228 -> [w360]
            tunnel: w227 -> [w359]
            tunnel: w226 -> [w356]
            tunnel: w225 -> [w355]
            tunnel: w224 -> [w354]
            tunnel: w223 -> [w358]
            tunnel: w222 -> [w357]
            tunnel: w221 -> [w353]
            tunnel: [w352] -> w204
            tunnel: w203 -> [w352]
            tunnel: w189 -> [w350]
            tunnel: [w350] -> w186
            tunnel: w185 -> [w351]
            tunnel: [w351] -> w182
            tunnel: w171 -> [w349]
            tunnel: w169 -> [w348]
            tunnel: w167 -> [w347]
            tunnel: w165 -> [w346]
            tunnel: [w349] -> w163
            tunnel: [w348] -> w159
            tunnel: [w347] -> w156
            tunnel: [w346] -> w155
            tunnel: w122 -> [w345]
            tunnel: w120 -> [w344]
            tunnel: [w345] -> w117
            tunnel: [w344] -> w115
            tunnel: w320 -> [w891]
            tunnel: [w891] -> w319
            tunnel: w318 -> [w890]
            tunnel: [w890] -> w317
            tunnel: w316 -> [w886]
            tunnel: [w886] -> w315
            tunnel: w314 -> [w887]
            tunnel: [w887] -> w313
            tunnel: [w887] -> w312
            tunnel: w311 -> [w889]
            tunnel: [w889] -> w310
            tunnel: w309 -> [w888]
            tunnel: [w888] -> w308
            tunnel: [w887] -> w305
            tunnel: [w887] -> w291
            tunnel: w276 -> [w885]
            tunnel: [w885] -> w274
            tunnel: w272 -> [w884]
            tunnel: [w884] -> w269
            tunnel: [w883] -> w253
            tunnel: w252 -> [w883]
            tunnel: [w882] -> w250
            tunnel: w249 -> [w882]
            tunnel: [w881] -> w248
            tunnel: w247 -> [w881]
            tunnel: [w880] -> w234
            tunnel: w233 -> [w880]
            tunnel: [w879] -> w205
            tunnel: w204 -> [w879]
            tunnel: [w878] -> w187
            tunnel: w186 -> [w878]
            tunnel: [w877] -> w183
            tunnel: w182 -> [w877]
            tunnel: w163 -> [w876]
            tunnel: [w876] -> w162
            tunnel: [w875] -> w160
            tunnel: w159 -> [w875]
            tunnel: [w874] -> w158
            tunnel: w156 -> [w874]
            tunnel: w155 -> [w873]
            tunnel: [w873] -> w154
            tunnel: [w872] -> w118
            tunnel: w117 -> [w872]
            tunnel: [w871] -> w116
            tunnel: w115 -> [w871]
            tunnel: [w912] -> w290
            tunnel: w319 -> [w941]
            tunnel: w317 -> [w940]
            tunnel: w315 -> [w937]
            tunnel: w313 -> [w936]
            tunnel: w312 -> [w935]
            tunnel: w310 -> [w925]
            tunnel: w308 -> [w924]
            tunnel: w305 -> [w926]
            tunnel: [w922] -> w289
            tunnel: [w923] -> w288
            tunnel: [w934] -> w287
            tunnel: [w933] -> w286
            tunnel: [w932] -> w285
            tunnel: [w931] -> w284
            tunnel: w291 -> [w921]
            tunnel: [w920] -> w283
            tunnel: [w919] -> w282
            tunnel: [w902] -> w281
            tunnel: [w918] -> w280
            tunnel: w274 -> [w917]
            tunnel: [w917] -> w273
            tunnel: [w916] -> w270
            tunnel: w269 -> [w916]
            tunnel: w253 -> [w915]
            tunnel: [w915] -> w251
            tunnel: w250 -> [w914]
            tunnel: w248 -> [w913]
            tunnel: [w914] -> w246
            tunnel: [w913] -> w245
            tunnel: w234 -> [w911]
            tunnel: [w907] -> w206
            tunnel: w205 -> [w907]
            tunnel: w187 -> [w905]
            tunnel: w183 -> [w904]
            tunnel: [w896] -> w181
            tunnel: [w902] -> w180
            tunnel: [w892] -> w179
            tunnel: [w901] -> w178
            tunnel: [w899] -> w177
            tunnel: [w897] -> w176
            tunnel: w162 -> [w900]
            tunnel: [w900] -> w161
            tunnel: w160 -> [w899]
            tunnel: w158 -> [w898]
            tunnel: [w898] -> w157
            tunnel: w154 -> [w897]
            tunnel: [w896] -> w132
            tunnel: [w892] -> w130
            tunnel: [w895] -> w127
            tunnel: w118 -> [w894]
            tunnel: w116 -> [w893]
            tunnel: w290 -> [w1137]
            tunnel: [w1134] -> w264
            tunnel: w289 -> [w1150]
            tunnel: [w1150] -> w263
            tunnel: w288 -> [w1149]
            tunnel: [w1149] -> w262
            tunnel: w287 -> [w1148]
            tunnel: [w1148] -> w261
            tunnel: w286 -> [w1147]
            tunnel: [w1147] -> w260
            tunnel: w285 -> [w1146]
            tunnel: [w1146] -> w259
            tunnel: w284 -> [w1145]
            tunnel: [w1145] -> w258
            tunnel: [w1138] -> w257
            tunnel: w283 -> [w1131]
            tunnel: w282 -> [w1139]
            tunnel: w281 -> [w1138]
            tunnel: w280 -> [w1140]
            tunnel: [w1137] -> w256
            tunnel: w273 -> [w1136]
            tunnel: w270 -> [w1135]
            tunnel: [w1133] -> w255
            tunnel: [w1121] -> w254
            tunnel: w251 -> [w1132]
            tunnel: w246 -> [w1129]
            tunnel: w245 -> [w1128]
            tunnel: [w1130] -> w242
            tunnel: [w1127] -> w239
            tunnel: [w1126] -> w236
            tunnel: [w1122] -> w235
            tunnel: [w1120] -> w207
            tunnel: w206 -> [w1120]
            tunnel: w181 -> [w1119]
            tunnel: w180 -> [w1118]
            tunnel: w179 -> [w1117]
            tunnel: w178 -> [w1116]
            tunnel: w177 -> [w1115]
            tunnel: w176 -> [w1113]
            tunnel: [w1111] -> w175
            tunnel: [w1110] -> w174
            tunnel: [w1109] -> w173
            tunnel: [w1108] -> w172
            tunnel: w161 -> [w1112]
            tunnel: w157 -> [w1114]
            tunnel: [w1111] -> w153
            tunnel: [w1110] -> w152
            tunnel: [w1109] -> w151
            tunnel: [w1108] -> w150
            tunnel: [w1107] -> w133
            tunnel: w132 -> [w1107]
            tunnel: [w1106] -> w131
            tunnel: w130 -> [w1106]
            tunnel: [w1105] -> w128
            tunnel: w127 -> [w1105]
            tunnel: w264 -> [w1182]
            tunnel: [w1189] -> w304
            tunnel: [w1188] -> w303
            tunnel: w263 -> [w1188]
            tunnel: [w1183] -> w300
            tunnel: w262 -> [w1183]
            tunnel: [w1187] -> w298
            tunnel: w261 -> [w1187]
            tunnel: [w1186] -> w296
            tunnel: w260 -> [w1186]
            tunnel: [w1185] -> w294
            tunnel: w259 -> [w1185]
            tunnel: [w1184] -> w292
            tunnel: w258 -> [w1184]
            tunnel: w257 -> [w1171]
            tunnel: w256 -> [w1172]
            tunnel: w255 -> [w1167]
            tunnel: [w1167] -> w267
            tunnel: w254 -> [w1173]
            tunnel: [w1173] -> w265
            tunnel: [w1175] -> w243
            tunnel: w242 -> [w1175]
            tunnel: [w1176] -> w240
            tunnel: w239 -> [w1176]
            tunnel: [w1177] -> w237
            tunnel: w236 -> [w1177]
            tunnel: w235 -> [w1181]
            tunnel: [w1170] -> w208
            tunnel: w207 -> [w1170]
            tunnel: w175 -> [w1166]
            tunnel: w174 -> [w1165]
            tunnel: w173 -> [w1164]
            tunnel: w172 -> [w1163]
            tunnel: w153 -> [w1162]
            tunnel: w152 -> [w1161]
            tunnel: w151 -> [w1160]
            tunnel: w150 -> [w1159]
            tunnel: [w1162] -> w148
            tunnel: [w1161] -> w146
            tunnel: [w1160] -> w144
            tunnel: [w1159] -> w142
            tunnel: w133 -> [w1158]
            tunnel: w131 -> [w1157]
            tunnel: [w1156] -> w129
            tunnel: w128 -> [w1156]
            tunnel: w304 -> [w1201]
            tunnel: w303 -> [w1216]
            tunnel: w300 -> [w1210]
            tunnel: w298 -> [w1215]
            tunnel: w296 -> [w1212]
            tunnel: w294 -> [w1214]
            tunnel: w292 -> [w1213]
            tunnel: w267 -> [w1206]
            tunnel: w265 -> [w1205]
            tunnel: w243 -> [w1204]
            tunnel: w240 -> [w1203]
            tunnel: w237 -> [w1202]
            tunnel: [w1195] -> w124
            tunnel: [w1216] -> w220
            tunnel: [w1210] -> w219
            tunnel: [w1215] -> w218
            tunnel: [w1212] -> w217
            tunnel: [w1214] -> w216
            tunnel: [w1213] -> w215
            tunnel: [w1206] -> w214
            tunnel: [w1205] -> w213
            tunnel: [w1204] -> w212
            tunnel: [w1203] -> w211
            tunnel: [w1202] -> w210
            tunnel: [w1200] -> w209
            tunnel: w208 -> [w1200]
            tunnel: [w1199] -> w149
            tunnel: w148 -> [w1199]
            tunnel: [w1198] -> w147
            tunnel: w146 -> [w1198]
            tunnel: [w1197] -> w145
            tunnel: w144 -> [w1197]
            tunnel: [w1196] -> w143
            tunnel: w142 -> [w1196]
            tunnel: w129 -> [w1194]
            tunnel: [w1193] -> w114
            tunnel: [w1192] -> w113
            tunnel: [w1191] -> w112
            tunnel: [w1190] -> w111
            tunnel: w220 -> [w1263]
            tunnel: w219 -> [w1262]
            tunnel: w218 -> [w1261]
            tunnel: w217 -> [w1260]
            tunnel: w216 -> [w1259]
            tunnel: w215 -> [w1258]
            tunnel: w214 -> [w1257]
            tunnel: w213 -> [w1256]
            tunnel: w212 -> [w1255]
            tunnel: w211 -> [w1254]
            tunnel: w210 -> [w1253]
            tunnel: w209 -> [w1246]
            tunnel: [w1263] -> w202
            tunnel: [w1262] -> w201
            tunnel: [w1261] -> w200
            tunnel: [w1260] -> w199
            tunnel: [w1259] -> w198
            tunnel: [w1258] -> w197
            tunnel: [w1257] -> w196
            tunnel: [w1256] -> w195
            tunnel: [w1255] -> w194
            tunnel: [w1254] -> w193
            tunnel: [w1253] -> w192
            tunnel: [w1246] -> w191
            tunnel: [w1245] -> w190
            tunnel: w149 -> [w1243]
            tunnel: w147 -> [w1242]
            tunnel: w145 -> [w1241]
            tunnel: w143 -> [w1240]
            tunnel: [w1243] -> w141
            tunnel: [w1242] -> w139
            tunnel: [w1241] -> w137
            tunnel: [w1240] -> w135
            tunnel: w114 -> [w1239]
            tunnel: w113 -> [w1238]
            tunnel: w112 -> [w1237]
            tunnel: w111 -> [w1236]
            tunnel: [w1231] -> w110
            tunnel: [w1274] -> w238
            tunnel: [w1275] -> w241
            tunnel: [w1276] -> w244
            tunnel: [w1277] -> w266
            tunnel: [w1278] -> w268
            tunnel: [w1279] -> w293
            tunnel: [w1280] -> w295
            tunnel: [w1281] -> w297
            tunnel: [w1282] -> w299
            tunnel: [w1283] -> w301
            tunnel: [w1284] -> w302
            tunnel: w202 -> [w1284]
            tunnel: w201 -> [w1283]
            tunnel: w200 -> [w1282]
            tunnel: w199 -> [w1281]
            tunnel: w198 -> [w1280]
            tunnel: w197 -> [w1279]
            tunnel: w196 -> [w1278]
            tunnel: w195 -> [w1277]
            tunnel: w194 -> [w1276]
            tunnel: w193 -> [w1275]
            tunnel: w192 -> [w1274]
            tunnel: w191 -> [w1270]
            tunnel: w190 -> [w1269]
            tunnel: [w1268] -> w140
            tunnel: w141 -> [w1268]
            tunnel: [w1267] -> w138
            tunnel: w139 -> [w1267]
            tunnel: [w1266] -> w136
            tunnel: w137 -> [w1266]
            tunnel: [w1265] -> w134
            tunnel: w135 -> [w1265]
            tunnel: [w1264] -> w126
            tunnel: w110 -> [w1264]
            frame #0 {
              n16 = Tick Count (ms)() -> (millisecond timer value=w332:u32)
            }
            frame #1 {
              n17 = while {
                tunnel: w364 -> [w371]
                tunnel: [w370] -> w363
                tunnel: [w369] -> w362
                tunnel: w350 -> [w367]
                stop <- w372 stop-if-true
                (unwired) "Daniel Schuster (geb. 20.03.1988)"
                n18 = event shown="[11] \"Write to File\": Value Change" {
                  selector: _ -> [_ _ _ _ _ _ _ _ _ _ _ _]
                  dyn-events: _ -> [_ _ _ _ _ _ _ _ _ _ _ _]
                  timeout: 1 -> [_ _ _ _ _ _ _ _ _ _ _ _]
                  tunnel: [TRUE ("Set Gauge to Zero") w380 w429 w450 w476 w511 w567 w618 w697 w768 "Set Gauge to Zero" _] -> w372
                  tunnel: w371 -> [w376 w379 w426 w448 w472 w510 w563 w616 w695 w766 w843 w865]
                  tunnel: [w375 w378 w425 w447 w474 w508 w565 w615 w694 w765 w842 w864] -> w370
                  tunnel: [w374 w377 w424 w446 w473 w509 w564 w614 w693 w764 w841 w863] -> w369
                  tunnel: w367 -> [_ _ _ _ _ _ _ _ _ _ w839 _]
                  event Timeout {
                    n19 = event-data() -> ()  [unwired: 1 in, 1 out]
                    n20 = Unbundle(w376) -> ("VISA resource name out"=w375:refnum<visa-resource-name>, "error out"=w374:errorcluster)  [unwired: 2 out]
                  }
                  event "Setpoint\n START": Value Change {
                    n21 = event-data() -> ()  [unwired: 1 in, 1 out]
                    n22 = stacked-sequence {
                      tunnel: w379 -> [_ w386 _]
                      tunnel: [_ w385 _] -> w377
                      tunnel: [_ w384 _] -> w378
                      frame #0 {
                        n23 = property on="Setpoint\n START" class="Bool"("Blinking"=TRUE) -> ()  [unwired: 2 in, 2 out]
                        n24 = property on="Read Temperature" class="Bool (strict)"("Blinking"=FALSE) -> ()  [unwired: 2 in, 2 out]
                      }
                      frame #1 {
                        n25 = for {
                          N: 2 -> [_]
                          tunnel: w386 -> [w390]
                          tunnel: [w389] -> w385
                          tunnel: [w388] -> w384
                          i -> [w392]
                          n26 = flat-sequence {
                            tunnel: [w395] -> w391
                            tunnel: w392 -> [w394]
                            tunnel: [w413] -> w393
                            tunnel: w391 -> [w412]
                            tunnel: w390 -> [w414]
                            tunnel: [w411] -> w389
                            tunnel: [w410] -> w388
                            tunnel: w393 -> [w420]
                            tunnel: w392 -> [w419]
                            frame #0 {
                              n27 = case shown="0, Default" w394 {
                                tunnel: [w404 w406] -> w395
                                frame 0, Default {
                                n28 = Multiply(x=10.0, y="SP 1 shall be (°C)") -> (x*y=w401:dbl)
                                n29 = local read "RAM"() -> (w399:bool)
                                n30 = Number To Hexadecimal String(1:i16 5 ("width (-)"), 2:w401) -> (0:w403:string)
                                n31 = Select(t="*P012", s=w399, f="*P012") -> (s? t:f=w396:string)
                                n32 = Concatenate Strings(w396, w403) -> (w404:string)
                                }
                                frame 1 {
                                n33 = local read "RAM"() -> (w409:bool)
                                n34 = Select(t="*G01", s=w409, f="*R01") -> (s? t:f=w406:string)
                                }
                              }
                            }
                            frame #1 {
                              n35 = Unbundle(w414) -> ("VISA resource name out"=w415:refnum<visa-resource-name>, "error out"=w417:errorcluster, "Delay (ms)"=w416:u32, "Write/\nRead"=w418:bool)
                              n36 = call "I3252_Comm_Interface.vi"("VISA resource name in"=w415, "error in"=w417, "Delay (ms)"=w416, "Write"=w418, "String to Write"=w412, "Read"=w418) -> ("VISA resource name out"=w410:refnum<visa-resource-name>, "error out"=w411:errorcluster, "Read String"=w413:string)  [unwired: 2 in]
                            }
                            frame #2 {
                              n37 = case shown="0, Default" w419 {
                                tunnel: w420 -> [_ w422]
                                frame 0, Default {
                                }
                                frame 1 {
                                n38 = call "I3252_Edit_Setpoint.vi"("Read String"=w422) -> ("Setpoint is"=→"SP 1 is (°C)":dbl)
                                }
                              }
                            }
                          }
                        }
                      }
                      frame #2 {
                        n39 = property on="Setpoint\n START" class="Bool"("Blinking"=FALSE) -> ()  [unwired: 2 in, 2 out]
                      }
                    }
                    n40 = Not(x="Setpoint\n START") -> (.not. x?=w380:bool)
                  }
                  event "Standby": Value Change {
                    n41 = event-data() -> ()  [unwired: 1 in, 1 out]
                    n42 = flat-sequence {
                      tunnel: [w437] -> w427
                      tunnel: w427 -> [w441]
                      tunnel: w426 -> [w440]
                      tunnel: [w439] -> w424
                      tunnel: [w438] -> w425
                      frame #0 {
                        n43 = local read "Standby"() -> (w430:bool)
                        n44 = Select(t=TRUE, s=w430, f=FALSE) -> (s? t:f=w433:bool)
                        n45 = property on="Standby" class="Bool (strict)"("Blinking"=w433) -> ()  [unwired: 2 in, 2 out]
                      }
                      frame #1 {
                        n46 = local read "Standby"() -> (w435:bool)
                        n47 = Select(t="*D03", s=w435, f="*E03") -> (s? t:f=w437:string)
                      }
                      frame #2 {
                        n48 = Unbundle(w440) -> ("VISA resource name out"=w442:refnum<visa-resource-name>, "error out"=w444:errorcluster, "Delay (ms)"=w443:u32, "Write/\nRead"=w445:bool)
                        n49 = call "I3252_Comm_Interface.vi"("VISA resource name in"=w442, "error in"=w444, "Delay (ms)"=w443, "Write"=w445, "String to Write"=w441, "Read"=w445) -> ("VISA resource name out"=w438:refnum<visa-resource-name>, "error out"=w439:errorcluster)  [unwired: 2 in, 1 out]
                      }
                    }
                    n50 = Not(x="Standby") -> (.not. x?=w429:bool)
                  }
                  event "Set Command": Value Change {
                    n51 = event-data() -> ()  [unwired: 1 in, 1 out]
                    n52 = stacked-sequence {
                      tunnel: w448 -> [_ w455 _]
                      tunnel: [_ w454 _] -> w447
                      tunnel: [_ w453 _] -> w446
                      frame #0 {
                        n53 = property on="Set Command" class="Bool"("Blinking"=TRUE) -> ()  [unwired: 2 in, 2 out]
                        n54 = property on="Read Temperature" class="Bool (strict)"("Blinking"=FALSE) -> ()  [unwired: 2 in, 2 out]
                      }
                      frame #1 {
                        n55 = flat-sequence {
                          tunnel: [w460] -> w457
                          tunnel: [w463] -> w456
                          tunnel: w457 -> [w464]
                          tunnel: w455 -> [w465]
                          tunnel: [w462] -> w454
                          tunnel: [w461] -> _
                          tunnel: [w461] -> w453
                          tunnel: w456 -> [w470]
                          frame #0 {
                            n56 = Concatenate Strings("*", "Command shall be") -> (w460:string)
                          }
                          frame #1 {
                            n57 = Unbundle(w465) -> ("VISA resource name out"=w469:refnum<visa-resource-name>, "error out"=w467:errorcluster, "Delay (ms)"=w468:u32, "Write/\nRead"=w466:bool)
                            n58 = call "I3252_Comm_Interface.vi"("VISA resource name in"=w469, "error in"=w467, "Delay (ms)"=w468, "Write"=w466, "String to Write"=w464, "Read"=w466) -> ("VISA resource name out"=w462:refnum<visa-resource-name>, "error out"=w461:errorcluster, "Read String"=w463:string)  [unwired: 2 in]
                          }
                          frame #2 {
                            "Command is" <- w470
                          }
                        }
                      }
                      frame #2 {
                        n59 = property on="Set Command" class="Bool"("Blinking"=FALSE) -> ()  [unwired: 2 in, 2 out]
                      }
                    }
                    n60 = Not(x="Set Command") -> (.not. x?=w450:bool)
                  }
                  event "Reset\nSTOPP": Value Change {
                    n61 = event-data() -> ()  [unwired: 1 in, 1 out]
                    n62 = stacked-sequence {
                      tunnel: [_ w483 _] -> w473
                      tunnel: [_ w482 _] -> w474
                      tunnel: w472 -> [_ w480 _]
                      frame #0 {
                        n63 = property on="Reset\nSTOPP" class="Bool"("Blinking"=TRUE) -> ()  [unwired: 2 in, 2 out]
                        n64 = property on="Read Temperature" class="Bool (strict)"("Blinking"=FALSE) -> ()  [unwired: 2 in, 2 out]
                      }
                      frame #1 {
                        n65 = for {
                          N: 2 -> [_]
                          tunnel: [w489] -> w483
                          tunnel: [w488] -> w482
                          tunnel: w480 -> [w487]
                          i -> [w485]
                          n66 = flat-sequence {
                            tunnel: w485 -> [w491]
                            tunnel: [w490] -> w486
                            tunnel: [w496] -> w489
                            tunnel: [w497] -> w488
                            tunnel: w487 -> [w498]
                            tunnel: w486 -> [w495]
                            tunnel: [w494] -> w484
                            tunnel: w485 -> [w504]
                            tunnel: w484 -> [w503]
                            frame #0 {
                              n67 = case shown="0, Default" w491 {
                                tunnel: ["*Z02" "*G01"] -> w490
                                frame 0, Default {
                                }
                                frame 1 {
                                }
                              }
                            }
                            frame #1 {
                              n68 = Unbundle(w498) -> ("VISA resource name out"=w499:refnum<visa-resource-name>, "error out"=w501:errorcluster, "Delay (ms)"=w500:u32, "Write/\nRead"=w502:bool)
                              n69 = call "I3252_Comm_Interface.vi"("VISA resource name in"=w499, "error in"=w501, "Delay (ms)"=w500, "Write"=w502, "String to Write"=w495, "Read"=w502) -> ("VISA resource name out"=w497:refnum<visa-resource-name>, "error out"=w496:errorcluster, "Read String"=w494:string)  [unwired: 2 in]
                            }
                            frame #2 {
                              n70 = case shown="0, Default" w504 {
                                tunnel: w503 -> [_ w506]
                                frame 0, Default {
                                }
                                frame 1 {
                                n71 = call "I3252_Edit_Setpoint.vi"("Read String"=w506) -> ("Setpoint is"=w505:dbl)
                                n72 = local write "SP 1 is (°C)"(w505) -> ()
                                }
                              }
                            }
                          }
                        }
                        n73 = Wait (ms)(milliseconds to wait=u32 4000) -> ()  [unwired: 1 out]
                      }
                      frame #2 {
                        n74 = property on="Reset\nSTOPP" class="Bool"("Blinking"=FALSE) -> ()  [unwired: 2 in, 2 out]
                      }
                    }
                    n75 = Not(x="Reset\nSTOPP") -> (.not. x?=w476:bool)
                  }
                  event "Auto Tune": Value Change {
                    n76 = event-data() -> ()  [unwired: 1 in, 1 out]
                    n77 = stacked-sequence {
                      tunnel: w510 -> [_ w517 w562]
                      tunnel: [_ w516 _] -> w509
                      tunnel: [_ w515 _] -> w508
                      frame #0 {
                        n78 = property on="Auto Tune" class="Bool"("Blinking"=TRUE) -> ()  [unwired: 2 in, 2 out]
                        n79 = property on="Read Temperature" class="Bool (strict)"("Blinking"=FALSE) -> ()  [unwired: 2 in, 2 out]
                      }
                      frame #1 {
                        n80 = for {
                          N: 4 -> [_]
                          tunnel: [w522] -> w515
                          tunnel: [w521] -> w516
                          tunnel: w517 -> [w520]
                          i -> [w525]
                          n81 = flat-sequence {
                            tunnel: w525 -> [w527]
                            tunnel: [w526] -> w523
                            tunnel: w523 -> [w542]
                            tunnel: [w541] -> w524
                            tunnel: [w544] -> w522
                            tunnel: [w543] -> w521
                            tunnel: w520 -> [w540]
                            tunnel: w525 -> [w550]
                            tunnel: w524 -> [w549]
                            frame #0 {
                              n82 = case shown="0, Default" w527 {
                                tunnel: ["*V01" w530 "*W0C35" "*Z02"] -> w526
                                frame 0, Default {
                                }
                                frame 1 {
                                n83 = local read "(°C)"() -> (w529:dbl)
                                n84 = Add(x=20.0, y=w529) -> (x+y=w536:dbl)
                                n85 = Multiply(x=10.0, y=w536) -> (x*y=w533:dbl)
                                n86 = Number To Hexadecimal String(1:i16 5 ("width (-)"), 2:w533) -> (0:w532:string)
                                n87 = Concatenate Strings("*W012", w532) -> (w530:string)
                                }
                                frame 2 {
                                # "35 hex = \n00110101 bin"
                                }
                                frame 3 {
                                }
                              }
                            }
                            frame #1 {
                              n88 = Unbundle(w540) -> ("VISA resource name out"=w548:refnum<visa-resource-name>, "error out"=w546:errorcluster, "Delay (ms)"=w547:u32, "Write/\nRead"=w545:bool)
                              n89 = call "I3252_Comm_Interface.vi"("VISA resource name in"=w548, "error in"=w546, "Delay (ms)"=w547, "Write"=w545, "String to Write"=w542, "Read"=w545) -> ("VISA resource name out"=w544:refnum<visa-resource-name>, "error out"=w543:errorcluster, "Read String"=w541:string)  [unwired: 2 in]
                            }
                            frame #2 {
                              n90 = case shown="0, Default" w550 {
                                tunnel: w549 -> [w552]
                                frame 0, Default {
                                n91 = call <vilib>:"Space Constant.vi"() -> ("String"=w555:string)
                                n92 = Search/Split String(string=w552, search string/char (-)=w555) -> (match + rest of string=w554:string)  [unwired: 1 in, 2 out]
                                n93 = Fract/Exp String To Number(use system decimal point (T)=FALSE, string=w554) -> (number=w551:dbl)  [unwired: 2 in, 1 out]
                                n94 = local write "(°C)"(w551) -> ()
                                }
                              }
                            }
                          }
                        }
                        n95 = Wait (ms)(milliseconds to wait=u32 45000) -> ()  [unwired: 1 out]
                      }
                      frame #2 {
                        n96 = Unbundle(w562) -> ("VISA resource name out"=w561:refnum<visa-resource-name>, "error out"=w559:errorcluster, "Delay (ms)"=w560:u32, "Write/\nRead"=w558:bool)
                        n97 = property on="Auto Tune" class="Bool"("Blinking"=FALSE) -> ()  [unwired: 2 in, 2 out]
                        n98 = call "I3252_Comm_Interface.vi"("VISA resource name in"=w561, "error in"=w559, "Delay (ms)"=w560, "Write"=w558, "String to Write"="*W01200000", "Read"=w558) -> ()  [unwired: 2 in, 3 out]
                      }
                    }
                    n99 = Not(x="Auto Tune") -> (.not. x?=w511:bool)
                  }
                  event "Write LOW/HI": Value Change {
                    n100 = event-data() -> ()  [unwired: 1 in, 1 out]
                    n101 = stacked-sequence {
                      tunnel: [_ w572 _] -> w565
                      tunnel: [_ w571 _] -> w564
                      tunnel: w563 -> [_ w570 _]
                      frame #0 {
                        n102 = property on="Write LOW/HI" class="Bool"("Blinking"=TRUE) -> ()  [unwired: 2 in, 2 out]
                        n103 = property on="Read Temperature" class="Bool (strict)"("Blinking"=FALSE) -> ()  [unwired: 2 in, 2 out]
                      }
                      frame #1 {
                        n104 = for {
                          N: 4 -> [_]
                          tunnel: [w576] -> w572
                          tunnel: [w575] -> w571
                          tunnel: w570 -> [w574]
                          i -> [w578]
                          n105 = flat-sequence {
                            tunnel: w578 -> [w580]
                            tunnel: [w581] -> w577
                            tunnel: w577 -> [w595]
                            tunnel: [w596] -> w579
                            tunnel: [w598] -> w576
                            tunnel: [w597] -> w575
                            tunnel: w574 -> [w594]
                            tunnel: w579 -> [w604]
                            tunnel: w578 -> [w603]
                            frame #0 {
                              n106 = case shown="1" w580 {
                                tunnel: [w583 w589 "*R27" "*R28"] -> w581
                                frame 0, Default {
                                n107 = Number To Hexadecimal String(1:i16 2 ("width (-)"), 2:"% LOW shall be") -> (0:w584:string)
                                n108 = Concatenate Strings("*W27", w584) -> (w583:string)
                                }
                                frame 1 {
                                n109 = Number To Hexadecimal String(1:i16 2 ("width (-)"), 2:"% High shall be") -> (0:w590:string)
                                n110 = Concatenate Strings("*W28", w590) -> (w589:string)
                                }
                                frame 2 {
                                }
                                frame 3 {
                                }
                              }
                            }
                            frame #1 {
                              n111 = Unbundle(w594) -> ("VISA resource name out"=w602:refnum<visa-resource-name>, "error out"=w600:errorcluster, "Delay (ms)"=w601:u32, "Write/\nRead"=w599:bool)
                              n112 = call "I3252_Comm_Interface.vi"("VISA resource name in"=w602, "error in"=w600, "Delay (ms)"=w601, "Write"=w599, "String to Write"=w595, "Read"=w599) -> ("VISA resource name out"=w598:refnum<visa-resource-name>, "error out"=w597:errorcluster, "Read String"=w596:string)  [unwired: 2 in]
                            }
                            frame #2 {
                              n113 = case shown="0, Default" w603 {
                                tunnel: w604 -> [_ w608 w612]
                                frame 0, Default {
                                }
                                frame 2 {
                                n114 = String Subset(string=w608, offset (0)=3) -> (substring=w606:string)  [unwired: 1 in]
                                n115 = Hexadecimal String To Number(string=w606) -> (number=→"% LOW is":u32)  [unwired: 2 in, 1 out]
                                }
                                frame 3 {
                                n116 = String Subset(string=w612, offset (0)=3) -> (substring=w610:string)  [unwired: 1 in]
                                n117 = Hexadecimal String To Number(string=w610) -> (number=→"% HIGH is":u32)  [unwired: 2 in, 1 out]
                                }
                              }
                            }
                          }
                        }
                      }
                      frame #2 {
                        n118 = property on="Write LOW/HI" class="Bool"("Blinking"=FALSE) -> ()  [unwired: 2 in, 2 out]
                      }
                    }
                    n119 = Not(x="Write LOW/HI") -> (.not. x?=w567:bool)
                  }
                  event "Set PID": Value Change {
                    n120 = event-data() -> ()  [unwired: 1 in, 1 out]
                    n121 = stacked-sequence {
                      tunnel: w616 -> [_ w623 _]
                      tunnel: [_ w622 _] -> w615
                      tunnel: [_ w621 _] -> w614
                      frame #0 {
                        n122 = property on="Set PID" class="Bool"("Blinking"=TRUE) -> ()  [unwired: 2 in, 2 out]
                        n123 = property on="Read Temperature" class="Bool (strict)"("Blinking"=FALSE) -> ()  [unwired: 2 in, 2 out]
                      }
                      frame #1 {
                        n124 = for {
                          N: 6 -> [_]
                          tunnel: w623 -> [w627]
                          tunnel: [w626] -> w622
                          tunnel: [w625] -> w621
                          i -> [w629]
                          n125 = flat-sequence {
                            tunnel: w629 -> [w631]
                            tunnel: [w632] -> w628
                            tunnel: w628 -> [w673]
                            tunnel: [w669] -> w630
                            tunnel: w627 -> [w672]
                            tunnel: [w671] -> w625
                            tunnel: [w670] -> w626
                            tunnel: w630 -> [w679]
                            tunnel: w629 -> [w678]
                            frame #0 {
                              n126 = case shown="0, Default" w631 {
                                tunnel: [w639 w647 w655 w657 w661 w665] -> w632
                                frame 0, Default {
                                n127 = local read "RAM"() -> (w633:bool)
                                n128 = Number To Hexadecimal String(1:i16 4 ("width (-)"), 2:"P (PB1) shall be") -> (0:w640:string)
                                n129 = Select(t="*P17", s=w633, f="*W17") -> (s? t:f=w634:string)
                                n130 = Concatenate Strings(w634, w640) -> (w639:string)
                                }
                                frame 1 {
                                n131 = local read "RAM"() -> (w641:bool)
                                n132 = Number To Hexadecimal String(1:i16 4 ("width (-)"), 2:"I ( Reset1) shall be") -> (0:w648:string)
                                n133 = Select(t="*P18", s=w641, f="*W18") -> (s? t:f=w643:string)
                                n134 = Concatenate Strings(w643, w648) -> (w647:string)
                                }
                                frame 2 {
                                n135 = local read "RAM"() -> (w650:bool)
                                n136 = Number To Hexadecimal String(1:i16 4 ("width (-)"), 2:"D (Rate) shall be") -> (0:w656:string)
                                n137 = Select(t="*P19", s=w650, f="*W19") -> (s? t:f=w651:string)
                                n138 = Concatenate Strings(w651, w656) -> (w655:string)
                                }
                                frame 3 {
                                n139 = local read "RAM"() -> (w660:bool)
                                n140 = Select(t="*G17", s=w660, f="*R17") -> (s? t:f=w657:string)
                                }
                                frame 4 {
                                n141 = local read "RAM"() -> (w664:bool)
                                n142 = Select(t="*G18", s=w664, f="*R18") -> (s? t:f=w661:string)
                                }
                                frame 5 {
                                n143 = local read "RAM"() -> (w668:bool)
                                n144 = Select(t="*G19", s=w668, f="*R19") -> (s? t:f=w665:string)
                                }
                              }
                            }
                            frame #1 {
                              n145 = Unbundle(w672) -> ("VISA resource name out"=w677:refnum<visa-resource-name>, "error out"=w675:errorcluster, "Delay (ms)"=w676:u32, "Write/\nRead"=w674:bool)
                              n146 = call "I3252_Comm_Interface.vi"("VISA resource name in"=w677, "error in"=w675, "Delay (ms)"=w676, "Write"=w674, "String to Write"=w673, "Read"=w674) -> ("VISA resource name out"=w670:refnum<visa-resource-name>, "error out"=w671:errorcluster, "Read String"=w669:string)  [unwired: 2 in]
                            }
                            frame #2 {
                              n147 = case shown="0, Default" w678 {
                                tunnel: w679 -> [_ w683 w687 w691]
                                frame 0, Default {
                                }
                                frame 3 {
                                n148 = String Subset(string=w683, offset (0)=3) -> (substring=w681:string)  [unwired: 1 in]
                                n149 = Hexadecimal String To Number(string=w681) -> (number=→"P (PB1) is":u32)  [unwired: 2 in, 1 out]
                                }
                                frame 4 {
                                n150 = String Subset(string=w687, offset (0)=3) -> (substring=w685:string)  [unwired: 1 in]
                                n151 = Hexadecimal String To Number(string=w685) -> (number=→"I ( Reset1) is":u32)  [unwired: 2 in, 1 out]
                                }
                                frame 5 {
                                n152 = String Subset(string=w691, offset (0)=3) -> (substring=w689:string)  [unwired: 1 in]
                                n153 = Hexadecimal String To Number(string=w689) -> (number=→"D (Rate) is":u32)  [unwired: 2 in, 1 out]
                                }
                              }
                            }
                          }
                        }
                      }
                      frame #2 {
                        n154 = property on="Set PID" class="Bool"("Blinking"=FALSE) -> ()  [unwired: 2 in, 2 out]
                      }
                    }
                    n155 = Not(x="Set PID") -> (.not. x?=w618:bool)
                  }
                  event "Get Values": Value Change {
                    n156 = event-data() -> ()  [unwired: 1 in, 1 out]
                    n157 = stacked-sequence {
                      tunnel: w695 -> [_ w702 _]
                      tunnel: [_ w701 _] -> w694
                      tunnel: [_ w700 _] -> w693
                      frame #0 {
                        n158 = property on="Get Values" class="Bool"("Blinking"=TRUE) -> ()  [unwired: 2 in, 2 out]
                        n159 = property on="Read Temperature" class="Bool (strict)"("Blinking"=FALSE) -> ()  [unwired: 2 in, 2 out]
                      }
                      frame #1 {
                        n160 = for {
                          N: 6 -> [_]
                          tunnel: w702 -> [w706]
                          tunnel: [w705] -> w701
                          tunnel: [w704] -> w700
                          i -> [w708]
                          n161 = flat-sequence {
                            tunnel: w708 -> [w710]
                            tunnel: [w711] -> w707
                            tunnel: w707 -> [w733]
                            tunnel: [w734] -> w709
                            tunnel: w706 -> [w732]
                            tunnel: [w731] -> w704
                            tunnel: [w730] -> w705
                            tunnel: w709 -> [w740]
                            tunnel: w708 -> [w739]
                            frame #0 {
                              n162 = case shown="0, Default" w710 {
                                tunnel: [w714 w718 w722 "*R27" "*R28" w728] -> w711
                                frame 0, Default {
                                n163 = local read "RAM"() -> (w715:bool)
                                n164 = Select(t="*G17", s=w715, f="*R17") -> (s? t:f=w714:string)
                                }
                                frame 1 {
                                n165 = local read "RAM"() -> (w719:bool)
                                n166 = Select(t="*G18", s=w719, f="*R18") -> (s? t:f=w718:string)
                                }
                                frame 2 {
                                n167 = local read "RAM"() -> (w723:bool)
                                n168 = Select(t="*G19", s=w723, f="*R19") -> (s? t:f=w722:string)
                                }
                                frame 3 {
                                }
                                frame 4 {
                                }
                                frame 5 {
                                n169 = local read "RAM"() -> (w729:bool)
                                n170 = Select(t="*G01", s=w729, f="*R01") -> (s? t:f=w728:string)
                                }
                              }
                            }
                            frame #1 {
                              n171 = Unbundle(w732) -> ("VISA resource name out"=w738:refnum<visa-resource-name>, "error out"=w736:errorcluster, "Delay (ms)"=w737:u32, "Write/\nRead"=w735:bool)
                              n172 = call "I3252_Comm_Interface.vi"("VISA resource name in"=w738, "error in"=w736, "Delay (ms)"=w737, "Write"=w735, "String to Write"=w733, "Read"=w735) -> ("VISA resource name out"=w730:refnum<visa-resource-name>, "error out"=w731:errorcluster, "Read String"=w734:string)  [unwired: 2 in]
                            }
                            frame #2 {
                              n173 = case shown="0, Default" w739 {
                                tunnel: w740 -> [w742 w746 w750 w754 w758 w762]
                                frame 0, Default {
                                n174 = String Subset(string=w742, offset (0)=3) -> (substring=w743:string)  [unwired: 1 in]
                                n175 = Hexadecimal String To Number(string=w743) -> (number=w741:u32)  [unwired: 2 in, 1 out]
                                n176 = local write "P (PB1) shall be"(w741) -> ()
                                n177 = local write "P (PB1) is"(w741) -> ()
                                }
                                frame 1 {
                                n178 = String Subset(string=w746, offset (0)=3) -> (substring=w747:string)  [unwired: 1 in]
                                n179 = Hexadecimal String To Number(string=w747) -> (number=w745:u32)  [unwired: 2 in, 1 out]
                                n180 = local write "I ( Reset1) shall be"(w745) -> ()
                                n181 = local write "I ( Reset1) is"(w745) -> ()
                                }
                                frame 2 {
                                n182 = String Subset(string=w750, offset (0)=3) -> (substring=w751:string)  [unwired: 1 in]
                                n183 = Hexadecimal String To Number(string=w751) -> (number=w749:u32)  [unwired: 2 in, 1 out]
                                n184 = local write "D (Rate) shall be"(w749) -> ()
                                n185 = local write "D (Rate) is"(w749) -> ()
                                }
                                frame 3 {
                                n186 = String Subset(string=w754, offset (0)=3) -> (substring=w755:string)  [unwired: 1 in]
                                n187 = Hexadecimal String To Number(string=w755) -> (number=w753:u32)  [unwired: 2 in, 1 out]
                                n188 = local write "% LOW shall be"(w753) -> ()
                                n189 = local write "% LOW is"(w753) -> ()
                                }
                                frame 4 {
                                n190 = String Subset(string=w758, offset (0)=3) -> (substring=w759:string)  [unwired: 1 in]
                                n191 = Hexadecimal String To Number(string=w759) -> (number=w757:u32)  [unwired: 2 in, 1 out]
                                n192 = local write "% High shall be"(w757) -> ()
                                n193 = local write "% HIGH is"(w757) -> ()
                                }
                                frame 5 {
                                n194 = call "I3252_Edit_Setpoint.vi"("Read String"=w762) -> ("Setpoint is"=w761:dbl)
                                n195 = local write "SP 1 is (°C)"(w761) -> ()
                                }
                              }
                            }
                          }
                        }
                      }
                      frame #2 {
                        n196 = property on="Get Values" class="Bool"("Blinking"=FALSE) -> ()  [unwired: 2 in, 2 out]
                      }
                    }
                    n197 = Not(x="Get Values") -> (.not. x?=w697:bool)
                  }
                  event "RAM": Value Change {
                    n198 = event-data() -> ()  [unwired: 1 in, 1 out]
                    n199 = stacked-sequence {
                      tunnel: w766 -> [_ w773 _]
                      tunnel: [_ w772 _] -> w765
                      tunnel: [_ w771 _] -> w764
                      frame #0 {
                        n200 = property on="RAM" class="Bool (strict)"("Blinking"=TRUE) -> ()  [unwired: 2 in, 2 out]
                        n201 = property on="Read Temperature" class="Bool (strict)"("Blinking"=FALSE) -> ()  [unwired: 2 in, 2 out]
                      }
                      frame #1 {
                        n202 = for {
                          N: 6 -> [_]
                          tunnel: w773 -> [w777]
                          tunnel: [w776] -> w772
                          tunnel: [w775] -> w771
                          i -> [w779]
                          n203 = flat-sequence {
                            tunnel: w779 -> [w781]
                            tunnel: [w782] -> w778
                            tunnel: w778 -> [w801]
                            tunnel: [w802] -> w780
                            tunnel: w777 -> [w805]
                            tunnel: [w804] -> w775
                            tunnel: [w803] -> w776
                            tunnel: w780 -> [w811]
                            tunnel: w779 -> [w810]
                            frame #0 {
                              n204 = case shown="0, Default" w781 {
                                tunnel: [w785 w789 w793 "*R27" "*R28" w799] -> w782
                                frame 0, Default {
                                n205 = local read "RAM"() -> (w786:bool)
                                n206 = Select(t="*G17", s=w786, f="*R17") -> (s? t:f=w785:string)
                                }
                                frame 1 {
                                n207 = local read "RAM"() -> (w790:bool)
                                n208 = Select(t="*G18", s=w790, f="*R18") -> (s? t:f=w789:string)
                                }
                                frame 2 {
                                n209 = local read "RAM"() -> (w794:bool)
                                n210 = Select(t="*G19", s=w794, f="*R19") -> (s? t:f=w793:string)
                                }
                                frame 3 {
                                }
                                frame 4 {
                                }
                                frame 5 {
                                n211 = local read "RAM"() -> (w800:bool)
                                n212 = Select(t="*G01", s=w800, f="*R01") -> (s? t:f=w799:string)
                                }
                              }
                            }
                            frame #1 {
                              n213 = Unbundle(w805) -> ("VISA resource name out"=w809:refnum<visa-resource-name>, "error out"=w807:errorcluster, "Delay (ms)"=w808:u32, "Write/\nRead"=w806:bool)
                              n214 = call "I3252_Comm_Interface.vi"("VISA resource name in"=w809, "error in"=w807, "Delay (ms)"=w808, "Write"=w806, "String to Write"=w801, "Read"=w806) -> ("VISA resource name out"=w803:refnum<visa-resource-name>, "error out"=w804:errorcluster, "Read String"=w802:string)  [unwired: 2 in]
                            }
                            frame #2 {
                              n215 = case shown="0, Default" w810 {
                                tunnel: w811 -> [w813 w817 w821 w825 w829 w833]
                                frame 0, Default {
                                n216 = String Subset(string=w813, offset (0)=3) -> (substring=w814:string)  [unwired: 1 in]
                                n217 = Hexadecimal String To Number(string=w814) -> (number=w812:u32)  [unwired: 2 in, 1 out]
                                n218 = local write "P (PB1) shall be"(w812) -> ()
                                n219 = local write "P (PB1) is"(w812) -> ()
                                }
                                frame 1 {
                                n220 = String Subset(string=w817, offset (0)=3) -> (substring=w818:string)  [unwired: 1 in]
                                n221 = Hexadecimal String To Number(string=w818) -> (number=w816:u32)  [unwired: 2 in, 1 out]
                                n222 = local write "I ( Reset1) shall be"(w816) -> ()
                                n223 = local write "I ( Reset1) is"(w816) -> ()
                                }
                                frame 2 {
                                n224 = String Subset(string=w821, offset (0)=3) -> (substring=w822:string)  [unwired: 1 in]
                                n225 = Hexadecimal String To Number(string=w822) -> (number=w820:u32)  [unwired: 2 in, 1 out]
                                n226 = local write "D (Rate) shall be"(w820) -> ()
                                n227 = local write "D (Rate) is"(w820) -> ()
                                }
                                frame 3 {
                                n228 = String Subset(string=w825, offset (0)=3) -> (substring=w826:string)  [unwired: 1 in]
                                n229 = Hexadecimal String To Number(string=w826) -> (number=w824:u32)  [unwired: 2 in, 1 out]
                                n230 = local write "% LOW shall be"(w824) -> ()
                                n231 = local write "% LOW is"(w824) -> ()
                                }
                                frame 4 {
                                n232 = String Subset(string=w829, offset (0)=3) -> (substring=w830:string)  [unwired: 1 in]
                                n233 = Hexadecimal String To Number(string=w830) -> (number=w828:u32)  [unwired: 2 in, 1 out]
                                n234 = local write "% High shall be"(w828) -> ()
                                n235 = local write "% HIGH is"(w828) -> ()
                                }
                                frame 5 {
                                n236 = call "I3252_Edit_Setpoint.vi"("Read String"=w833) -> ("Setpoint is"=w832:dbl)
                                n237 = local write "SP 1 is (°C)"(w832) -> ()
                                }
                              }
                            }
                          }
                        }
                      }
                      frame #2 {
                        n238 = property on="RAM" class="Bool (strict)"("Blinking"=FALSE) -> ()  [unwired: 2 in, 2 out]
                      }
                    }
                    n239 = Not(x="RAM") -> (.not. x?=w768:bool)
                  }
                  event "Set Gauge to Zero": Value Change {
                    n240 = event-data() -> ()  [unwired: 1 in, 1 out]
                    n241 = flat-sequence {
                      tunnel: w839 -> [w844]
                      tunnel: [w844] -> w838
                      tunnel: w838 -> [w846]
                      tunnel: [w850] -> w837
                      tunnel: [w849] -> w836
                      tunnel: [w846] -> w835
                      tunnel: w837 -> [w856]
                      tunnel: w836 -> [w855]
                      tunnel: w835 -> [w851]
                      frame #0 {
                        n242 = property on="Set Gauge to Zero" class="Bool"("Blinking"=TRUE) -> ()  [unwired: 2 in, 2 out]
                      }
                      frame #1 {
                        w847 = 0 items=["sensor 1", "sensor 2", "test"] ("Sensor Nr.:")
                        n243 = call "DUAL GAUGE-Get Pressure,Status.vi"("Sensor Nr.:"=w847, "Referenz in"=w846) -> ("Pressure"=w850:dbl)  [unwired: 6 in, 3 out]
                        "Pressure 2 (mbar)" <- w850
                        n244 = call "DUAL GAUGE-Offset display.vi"("W/R"=FALSE, "Referenz in"=w846) -> ("Sensor 1 Get"=w849:dbl)  [unwired: 6 in, 3 out]
                        "Old Offset (mbar)" <- w849
                      }
                      frame #2 {
                        n245 = Add(x=w856, y=w855) -> (x+y=w852:dbl)
                        n246 = call "DUAL GAUGE-Offset display.vi"("W/R"=TRUE, "Sensor 1 Set"=w852, "Referenz in"=w851) -> ("Sensor 1 Get"=→"Current Offset (mbar)":dbl)  [unwired: 5 in, 3 out]
                      }
                      frame #3 {
                        n247 = property on="Set Gauge to Zero" class="Bool"("Blinking"=TRUE) -> ()  [unwired: 2 in, 2 out]
                      }
                    }
                    n248 = Unbundle(w843) -> ("VISA resource name out"=w842:refnum<visa-resource-name>, "error out"=w841:errorcluster)  [unwired: 2 out]
                  }
                  event "Write to File": Value Change {
                    n249 = event-data() -> ("NewVal"=w862:bool)  [unwired: 1 in]
                    n250 = Unbundle(w865) -> ("VISA resource name out"=w864:refnum<visa-resource-name>, "error out"=w863:errorcluster)  [unwired: 2 out]
                    n251 = local read "File Path"() -> (w858:path)
                    n252 = case shown="True" w862 {
                      tunnel: w858 -> [_ w870]
                      tunnel: "User" -> [_ w869]
                      tunnel: "Sample" -> [_ w868]
                      tunnel: [path "" ("File Path") w867] -> w859
                      frame False {
                      }
                      frame True {
                        n253 = call "Header.vi"("Sample"=w868, "User"=w869, "File Path"=w870) -> ("File Path"=w867:path)
                      }
                    }
                    n254 = local write "File Path"(w859) -> ()
                  }
                }
              }
              n255 = Bundle(cluster=w364, "VISA resource name out"=w363, "error out"=w362) -> (w361:T7)  [unwired: 2 in]
            }
            frame #2 {
            }
            frame #3 {
              (unwired) "Daniel Schuster (geb. 20.03.1988)"
              n256 = node-c288(w936) -> (w939:T3)  [unwired: 2 in]
              n257 = node-c288(w926) -> (w928:T3)  [unwired: 2 in]
              n258 = node-c288(w921) -> (w930:T3)  [unwired: 2 in]
              n259 = node-c288(w935) -> (w943:T3)  [unwired: 2 in]
              n260 = timed-sequence {
                timing: w939 -> [_]
                timing-out: [_] -> w938
                tunnel: w937 -> [w1040]
                tunnel: [w1039] -> w932
                tunnel: [w1038] -> w931
                tunnel: [w1037] -> w918
                n261 = timed-flat-sequence {
                  tunnel: w1040 -> [w1044]
                  tunnel: [w1043] -> w1039
                  tunnel: [w1042] -> w1038
                  tunnel: [w1041] -> w1037
                  n262 = node-c288() -> ()  [unwired: 1 in, 1 out]
                  n263 = case shown="True" "Read Temperature" {
                    tunnel: w1044 -> [w1048 w1053]
                    tunnel: [w1047 w1052] -> w1043
                    tunnel: [w1046 w1051] -> w1042
                    tunnel: [_ w1050] -> w1041
                    frame False {
                      n264 = Unbundle(w1048) -> ("VISA resource name out"=w1047:refnum<visa-resource-name>, "error out"=w1046:errorcluster)  [unwired: 2 out]
                      n265 = property on="Read Temperature" class="Bool (strict)"("Blinking"=FALSE) -> ()  [unwired: 2 in, 2 out]
                    }
                    frame True {
                      n266 = stacked-sequence {
                        tunnel: w1053 -> [_ w1058]
                        tunnel: [_ w1057] -> w1052
                        tunnel: [_ w1056] -> w1051
                        tunnel: [_ w1055] -> w1050
                        frame #0 {
                          n267 = property on="Read Temperature" class="Bool (strict)"("Blinking"=TRUE) -> ()  [unwired: 2 in, 2 out]
                        }
                        frame #1 {
                          n268 = Unbundle(w1058) -> ("VISA resource name out"=w1062:refnum<visa-resource-name>, "error out"=w1060:errorcluster, "Delay (ms)"=w1061:u32, "Write/\nRead"=w1059:bool)
                          n269 = call "I3252_Comm_Interface.vi"("VISA resource name in"=w1062, "error in"=w1060, "Delay (ms)"=w1061, "Write"=w1059, "String to Write"="*V01", "Read"=w1059) -> ("VISA resource name out"=w1057:refnum<visa-resource-name>, "error out"=w1056:errorcluster, "Read String"=w1055:string)  [unwired: 2 in]
                        }
                      }
                    }
                  }
                  n270 = node-c288() -> ()  [unwired: 1 in, 1 out]
                }
              }
              n271 = timed-sequence {
                timing: w928 -> [_]
                timing-out: [_] -> w927
                tunnel: w925 -> [w948]
                tunnel: w924 -> [w947]
                tunnel: [w946] -> w922
                tunnel: [w945] -> w923
                tunnel: [w944] -> w919
                n272 = timed-flat-sequence {
                  tunnel: w948 -> [w953]
                  tunnel: w947 -> [w952]
                  tunnel: [w951] -> w946
                  tunnel: [w950] -> w945
                  tunnel: [w949] -> w944
                  n273 = node-c288() -> ()  [unwired: 1 in, 1 out]
                  n274 = case shown="False" "Read VC 840 2" {
                    tunnel: w953 -> [w957 w963]
                    tunnel: w952 -> [w958 w962]
                    tunnel: [w957 w961] -> w951
                    tunnel: [w958 w960] -> w950
                    tunnel: [0.0 ("Reading") w959] -> w949
                    frame False {
                      n275 = property on="Read VC 840 2" class="Bool (strict)"("Blinking"=FALSE) -> ()  [unwired: 2 in, 2 out]
                    }
                    frame True {
                      n276 = stacked-sequence {
                        tunnel: w963 -> [_ w970]
                        tunnel: w962 -> [_ w969]
                        tunnel: [_ w968] -> w961
                        tunnel: [_ w967] -> w960
                        tunnel: [_ w965] -> w959
                        frame #0 {
                          n277 = property on="Read VC 840 2" class="Bool (strict)"("Blinking"=TRUE) -> ()  [unwired: 2 in, 2 out]
                        }
                        frame #1 {
                          n278 = call "VC840_Read.vi"("error in (no error)"=w969, "VISA resource name"=w970) -> ("error out"=w967:errorcluster, "Unit"=→"Unit 2":string, "Reading"=w965:dbl, "VISA resource name out"=w968:refnum<visa-resource-name>, "Status"=→"Status 2":T2, "Mode"=→"Mode 2":enum16{"?", "Diode", "Beep", "DC", "AC"})  [unwired: 4 out]
                          "Reading 2" <- w965
                        }
                      }
                    }
                  }
                  n279 = node-c288() -> ()  [unwired: 1 in, 1 out]
                }
              }
              n280 = timed-sequence {
                timing: w930 -> [_]
                timing-out: [_] -> w929
                tunnel: w905 -> [w984]
                tunnel: w904 -> [w983]
                tunnel: [w982] -> w903
                tunnel: [w981] -> w895
                tunnel: w894 -> [w980]
                tunnel: w893 -> [w979]
                n281 = timed-flat-sequence {
                  tunnel: w984 -> [w990]
                  tunnel: w983 -> [w989]
                  tunnel: [w988] -> w982
                  tunnel: [w987] -> w981
                  tunnel: w980 -> [w986]
                  tunnel: w979 -> [w985]
                  n282 = node-c288() -> ()  [unwired: 1 in, 1 out]
                  n283 = case shown="True" "Read Pressure" {
                    tunnel: w990 -> [w996 w1005]
                    tunnel: w989 -> [w995 w1004]
                    tunnel: [w998 w1003] -> w988
                    tunnel: [w994 w1002] -> w987
                    tunnel: w986 -> [w993 w1001]
                    tunnel: w985 -> [w992 w1000]
                    frame False {
                      w997 = 0.0 ("Pressure")
                      n284 = property on="Read Pressure" class="Bool (strict)"("Blinking"=FALSE) -> ()  [unwired: 2 in, 2 out]
                      n285 = Bundle("Pressure"=w997, "Pressure"=w997, "Pressure"=w997, "Pressure"=w997) -> (w998:T8)  [unwired: 1 in]
                      n286 = Bundle("COM5 in"=w996, "error out"=w993, "COM6 in"=w995, "error out"=w992) -> (w994:T9)  [unwired: 1 in]
                    }
                    frame True {
                      n287 = stacked-sequence {
                        tunnel: w1005 -> [_ w1030]
                        tunnel: w1004 -> [_ w1029]
                        tunnel: [_ w1021] -> w1003
                        tunnel: [_ w1013] -> w1002
                        tunnel: w1001 -> [_ w1008]
                        tunnel: w1000 -> [_ w1007]
                        frame #0 {
                          n288 = property on="Read Pressure" class="Bool (strict)"("Blinking"=TRUE) -> ()  [unwired: 2 in, 2 out]
                        }
                        frame #1 {
                          n289 = call "PresureGetSubVI.vi"("COM5 in"=w1030, "Fehler (Eingang)"=w1008, "COM6 in"=w1029, "Fehler (Eingang) 2"=w1007) -> ("Status Baratron"=→"Status Baratron":i32, "Status Pirani"=→"Status Pirani":i32, "Status FullRange"=→"Status FullRange":i32, "Status Sensor 4"=→"Status Sensor 4":i32, "COM5 out"=w1015:refnum<visa-resource-name>, "COM6 out"=w1014:refnum<visa-resource-name>, "Pressure Baratron"=w1016:dbl, "Pressure FullRange"=w1022:dbl, "Cluster (Ausgang)"=w1010:errorcluster, "Pressure Pirani"=w1024:dbl, "Pressure Sensor 4"=w1023:dbl, "Cluster (Ausgang) 2"=w1009:errorcluster)  [unwired: 4 in]
                          "Pressure Baratron" <- w1016
                          "Pressure FullRange" <- w1022
                          "Pressure OpenPort" <- w1023
                          "Pressure Pirani" <- w1024
                          "Current Baratron (mbar)" <- w1016
                          n290 = Unbundle(w1009) -> ("status"=w1011:bool, "code"=w1018:i32)  [unwired: 1 out]
                          n291 = Bundle("COM5 out"=w1015, "Cluster (Ausgang)"=w1010, "COM6 out"=w1014, "Cluster (Ausgang) 2"=w1009) -> (w1013:T10)  [unwired: 1 in]
                          n292 = Unbundle(w1010) -> ("status"=w1012:bool, "code"=w1020:i32)  [unwired: 1 out]
                          n293 = Bundle("status"=w1012, "code"=w1020) -> (→"Error COM5 Out":cluster{"status":bool, "code":i32})  [unwired: 1 in]
                          n294 = Bundle("status"=w1011, "code"=w1018) -> (→"Error COM6 Out":cluster{"status":bool, "code":i32})  [unwired: 1 in]
                          n295 = Bundle("Pressure Baratron"=w1016, "Pressure FullRange"=w1022, "Pressure Pirani"=w1024, "Pressure Sensor 4"=w1023) -> (w1021:T11)  [unwired: 1 in]
                        }
                      }
                    }
                  }
                  n296 = node-c288() -> ()  [unwired: 1 in, 1 out]
                }
              }
              n297 = timed-sequence {
                timing: w943 -> [_]
                timing-out: [_] -> w942
                tunnel: w941 -> [w1074]
                tunnel: w940 -> [w1073]
                tunnel: [w1072] -> w934
                tunnel: [w1071] -> w933
                tunnel: [w1070] -> w920
                n298 = timed-flat-sequence {
                  tunnel: w1074 -> [w1079]
                  tunnel: w1073 -> [w1078]
                  tunnel: [w1077] -> w1072
                  tunnel: [w1076] -> w1071
                  tunnel: [w1075] -> w1070
                  n299 = node-c288() -> ()  [unwired: 1 in, 1 out]
                  n300 = case shown="True" "Read VC 840 1" {
                    tunnel: w1079 -> [w1083 w1089]
                    tunnel: w1078 -> [w1084 w1088]
                    tunnel: [w1083 w1087] -> w1077
                    tunnel: [w1084 w1086] -> w1076
                    tunnel: [0.0 ("Reading") w1085] -> w1075
                    frame False {
                      n301 = property on="Read VC 840 1" class="Bool (strict)"("Blinking"=FALSE) -> ()  [unwired: 2 in, 2 out]
                    }
                    frame True {
                      n302 = stacked-sequence {
                        tunnel: w1089 -> [_ w1096]
                        tunnel: w1088 -> [_ w1095]
                        tunnel: [_ w1094] -> w1087
                        tunnel: [_ w1093] -> w1086
                        tunnel: [_ w1091] -> w1085
                        frame #0 {
                          n303 = property on="Read VC 840 1" class="Bool (strict)"("Blinking"=TRUE) -> ()  [unwired: 2 in, 2 out]
                        }
                        frame #1 {
                          n304 = call "VC840_Read.vi"("error in (no error)"=w1095, "VISA resource name"=w1096) -> ("error out"=w1093:errorcluster, "Unit"=→"Unit 1":string, "Reading"=w1091:dbl, "VISA resource name out"=w1094:refnum<visa-resource-name>, "Status"=→"Status 1":T2, "Mode"=→"Mode 1":enum16{"?", "Diode", "Beep", "DC", "AC"})  [unwired: 4 out]
                          "Reading 1" <- w1091
                        }
                      }
                    }
                  }
                  n305 = node-c288() -> ()  [unwired: 1 in, 1 out]
                }
              }
              n306 = Tick Count (ms)() -> (millisecond timer value=w906:u32)
              n307 = Subtract(x=w906, y=w911) -> (x-y=w910:u32)
              n308 = Divide(x=w910, y=u32 1000) -> (x/y=w908:dbl)
              n309 = node-c288(w942) -> ()  [unwired: 1 out]
              n310 = node-c288(w927) -> ()  [unwired: 1 out]
              n311 = node-c288(w938) -> ()  [unwired: 1 out]
              n312 = To Double Precision Float(number=w908) -> (double precision float=w912:dbl)
              "current time (s)" <- w912
              n313 = node-c288(w929) -> ()  [unwired: 1 out]
              n314 = Unbundle(w903) -> ("Pressure Baratron"=w902:dbl, "Pressure FullRange"=w896:dbl, "Pressure Pirani"=w892:dbl, "Pressure Sensor 4"=w901:dbl)
              "Pressure Baratron 2" <- w902
              "Pressure FullRange 2" <- w896
              "Pressure OpenPort2" <- w901
              "Pressure Pirani 2" <- w892
            }
            frame #4 {
              n315 = Build Array (concatenate)(w1112, w1118) -> (w1111:dbl[])
              n316 = Build Array (concatenate)(w1115, w1119) -> (w1110:dbl[])
              n317 = Build Array (concatenate)(w1114, w1117) -> (w1109:dbl[])
              n318 = Build Array (concatenate)(w1113, w1116) -> (w1108:dbl[])
              n319 = Greater?(x=w1138, y="Pressure Limit (mbar)") -> (0:w1141:bool)
              n320 = case shown="False" w1141 {
                frame False {
                  n321 = property on="Standby" class="Bool (strict)"("DisabledEnum"=T6."Enabled" ("Disabled")) -> ()  [unwired: 2 in, 2 out]
                }
                frame True {
                  n322 = property on="Standby" class="Bool (strict)"("Val(Sgnl)"=TRUE ("Standby"), "DisabledEnum"=T6."Disabled" ("Disabled")) -> ()  [unwired: 2 in, 2 out]
                }
              }
              n323 = call "Resistivity_Calculation.vi"("Reading 1 (V)"=w1131, "Constant"="Constant", "Thickness (nm)"="Thickness (nm)", "Reading 2 (A)"=w1139) -> ("Resivtivity (Ohm*cm)"=w1123:dbl, "Current"=w1124:dbl, "Voltage"=w1125:dbl)
              "Resistivity (Ohm*cm)" <- w1123
              "Voltage (V)" <- w1125
              "Current (A)" <- w1124
              n324 = call "I3252_Edit_Temperature.vi"("Temp. String"=w1140) -> ("Temp. (°C)"=w1134:dbl)
              "(°C)" <- w1134
              n325 = Build Array (concatenate)(w1136, w1137) -> (w1133:dbl[])
              n326 = Build Array (concatenate)(w1135, w1134) -> (w1121:dbl[])
              n327 = Build Array (concatenate)(w1132, w1125) -> (w1130:dbl[])
              n328 = Build Array (concatenate)(w1129, w1124) -> (w1127:dbl[])
              n329 = Build Array (concatenate)(w1128, w1123) -> (w1126:dbl[])
              n330 = Build Array(w1125, w1124, w1123) -> (w1122:dbl[])
            }
            frame #5 {
              n331 = Bundle(w1167, w1166) -> (→"CMR275 Baratron":cluster{dbl[], dbl[]})  [unwired: 1 in]
              n332 = Bundle(w1167, w1165) -> (→"PKR251 FullRange":cluster{dbl[], dbl[]})  [unwired: 1 in]
              n333 = Bundle(w1167, w1164) -> (→"Pirani (VVP1 Scroll)":cluster{dbl[], dbl[]})  [unwired: 1 in]
              n334 = Bundle(w1167, w1163) -> (→"Pressure OpenPort":cluster{dbl[], dbl[]})  [unwired: 1 in]
              n335 = Bundle(w1167, w1173) -> (→"Thermocouple (Sample holder 1)":cluster{dbl[], dbl[]})  [unwired: 1 in]
              n336 = Bundle(w1167, w1175) -> (→"Voltage":cluster{dbl[], dbl[]})  [unwired: 1 in]
              n337 = Bundle(w1167, w1176) -> (→"Current":cluster{dbl[], dbl[]})  [unwired: 1 in]
              n338 = Bundle(w1167, w1177) -> (→"Resistivity":cluster{dbl[], dbl[]})  [unwired: 1 in]
              n339 = Build Array (concatenate)(w1172, w1182, w1181, w1171, w1158, w1157) -> (w1189:dbl[])
              "appended array" <- w1189
            }
            frame #6 {
              n340 = Unbundle(w1194) -> ("COM5 out"=w1193:refnum<visa-resource-name>, "Cluster (Ausgang)"=w1192:errorcluster, "COM6 out"=w1191:refnum<visa-resource-name>, "Cluster (Ausgang) 2"=w1190:errorcluster)
              n341 = case shown="True" "Write to File" {
                tunnel: [_ w1222] -> w1208
                tunnel: "File Path" -> [_ w1220]
                tunnel: w1201 -> [_ w1218]
                frame False {
                  n342 = property on="Write to File" class="Bool (strict)"("Blinking"=FALSE) -> ()  [unwired: 2 in, 2 out]
                }
                frame True {
                  n343 = flat-sequence {
                    tunnel: [w1224] -> w1221
                    tunnel: w1220 -> [w1224]
                    tunnel: [w1223] -> w1219
                    tunnel: w1218 -> [w1223]
                    tunnel: [w1229] -> w1222
                    tunnel: w1221 -> [w1228]
                    tunnel: w1219 -> [w1227]
                    frame #0 {
                      n344 = property on="Write to File" class="Bool (strict)"("Blinking"=TRUE) -> ()  [unwired: 2 in, 2 out]
                    }
                    frame #1 {
                      n345 = call-poly <vilib>:"Write To Spreadsheet File.vi"("format (%.3f)"="%g", "append to file? (new file:F)"=TRUE ("transpose? (no:F)"), "1D data"=w1227, "file path (dialog if empty)"=w1228) -> ("new file path (Not A Path if cancelled)"=w1229:path)  [unwired: 4 in]
                    }
                  }
                }
              }
              n346 = Merge Errors(w1213, w1212, w1210, w1192, w1190) -> (w1211:errorcluster)
              n347 = call <vilib>:"Simple Error Handler.vi"("error in (no error)"=w1211) -> ("error?"=w1195:bool)  [unwired: 4 in, 4 out]
              n348 = local write "File Path"(w1208) -> ()
            }
            frame #7 {
              w1245 = u32 1000 ("y")
              n349 = Tick Count (ms)() -> (millisecond timer value=w1247:u32)
              n350 = Subtract(x=w1247, y=w1246) -> (x-y=w1248:u32)
              n351 = VISA Flush I/O Buffer(VISA resource name=w1239, error in (no error)=w1238) -> (VISA resource name out=w1234:refnum<visa-resource-name>, error out=w1235:errorcluster)  [unwired: 1 in]
              n352 = VISA Flush I/O Buffer(VISA resource name=w1237, error in (no error)=w1236) -> (VISA resource name out=w1233:refnum<visa-resource-name>, error out=w1232:errorcluster)  [unwired: 1 in]
              n353 = Divide(x=w1248, y=w1245) -> (x/y=→"loop time (s)":dbl)
              n354 = Subtract(x="Intervall (s)", y=u32 1) -> (x-y=w1249:u32)
              n355 = Multiply(x=w1249, y=w1245) -> (x*y=w1252:u32)
              n356 = Wait (ms)(milliseconds to wait=w1252) -> ()  [unwired: 1 out]
              n357 = Bundle("COM5 out"=w1234, "error out"=w1235, "COM6 out"=w1233, "error out"=w1232) -> (w1231:T12)  [unwired: 1 in]
            }
            frame #8 {
              n358 = Tick Count (ms)() -> (millisecond timer value=w1272:u32)
              n359 = Subtract(x=w1272, y=w1270) -> (x-y=w1271:u32)
              n360 = Divide(x=w1271, y=w1269) -> (x/y=→"data logger intervall (s)":dbl)
            }
          }
          n361 = Exclusive Or(1:"stop", 2:w124) -> (0:w125:bool)
        }
      }
      frame #4 {
        n362 = call "VC840_Close.vi"("error in (no error)"=w1291, "VISA resource name"=w1292) -> ("error out"=w1300:errorcluster)  [unwired: 9 in]
        n363 = call "VC840_Close.vi"("error in (no error)"=w1293, "VISA resource name"=w1294) -> ("error out"=w1298:errorcluster)  [unwired: 9 in]
        n364 = VISA Close(VISA resource name=w1296, error in (no error)=w1295) -> (error out=w1297:errorcluster)
        n365 = Unbundle(w1289) -> ("COM5 out"=w1288:refnum<visa-resource-name>, "error out"=w1287:errorcluster, "COM6 out"=w1285:refnum<visa-resource-name>, "error out"=w1286:errorcluster)
        n366 = VISA Close(VISA resource name=w1288, error in (no error)=w1287) -> ()  [unwired: 1 out]
        n367 = VISA Close(VISA resource name=w1285, error in (no error)=w1286) -> ()  [unwired: 1 out]
        n368 = Merge Errors(w1297, w1298, w1300) -> (w1299:errorcluster)
        n369 = call <vilib>:"Simple Error Handler.vi"("error in (no error)"=w1299) -> ("error?"=w1290:bool)  [unwired: 1 in, 7 out]
        n370 = Stop(stop? (T)=w1290) -> ()
      }
    }
  }
